vi "Dashboard Main.vi"() -> ()   [LabVIEW 2014]
uses:
  <vilib>/Rock Robotics/WPI/Dashboard/WPI_DashboardLogging Global.vi
  <vilib>/Utility/config.llb/NI_LVConfig.lvlib
  <vilib>/Utility/config.llb/Write Key (I32).vi
  Common Code/Utilities/PDP Data.ctl
  Common Code/commandCluster.ctl
  Common Code/AutonomousDBPacket.ctl
  Common Code/Roller Mode Enum.ctl
  Common Code/Auto Roller Commands.ctl
  Common Code/Roller Indicators.ctl
  Common Code/Elevator State.ctl
  Common Code/Elevator Status.ctl
  Common Code/Dashboard Display Data.ctl
  <vilib>/Utility/miscctls.llb/LVPointTypeDef.ctl
  Common Code/IMU Data.ctl
  Common Code/Inner Roller States.ctl
  Common Code/Elevator Mode.ctl
  Common Code/Encoder Values.ctl
  Common Code/Encoder Values SuperCluster.ctl
  Common Code/Utilities/PCM Data.ctl
  Common Code/Power and Diagnostic Data.ctl
  Common Code/Loop Timings.ctl
  Common Code/Ultrasonic Indicators.ctl
  Robot Code/Sensors/Pot Data.ctl
  Robot Code/Drivetrain Code/Drivetrain Mode.ctl
  Common Code/Drivetrain Status.ctl
  Robot Code/Rollers/ThinRollerIndicators.ctl
  Common Code/Auto Elevator Indicators.ctl
  Common Code/Dist Drive Status.ctl
  Common Code/Drivetrain Settings.ctl
  Common Code/Encoder Control.ctl
  Common Code/Elevator Presets.ctl
  Common Code/Elevator DB Control.ctl
  Common Code/Roller Control.ctl
  Common Code/Dashboard Control Data.ctl
  navX-MXP Library/COMMON/TypeDefs/Value TypeDefs/navX NAVX_OP_STATUS.ctl
  navX-MXP Library/navX-MXP IMU.lvlib
  navX-MXP Library/COMMON/TypeDefs/Value TypeDefs/navX NAVX_CAL_STATUS.ctl
  Robot Code/Rollers/Untip Can States.ctl
  Common Code/Yaw Rate Compensation Indicators.ctl
  Robot Code/Pike/Pike DB Controls.ctl
  Robot Code/Pike/Pike Mode.ctl
  Robot Code/Pike/Pike State.ctl
  Robot Code/Pike/Pike Indicators.ctl
  Common Code/Elevator Idle Mode.ctl
  Robot Code/Elevator/Elevator Command.ctl
  Robot Code/Elevator/Elevator Control Command.ctl
  <vilib>/Utility/inputDevices.llb/keyboardAcquire.vi
  <vilib>/Utility/config.llb/Write Key (String).vi
  <vilib>/Rock Robotics/WPI/Camera/WPI_CameraImageSize.ctl
  <vilib>/Rock Robotics/WPI/Camera/WPI_CameraSettings Read MJPG.ctl
  Vision/Particle Filter Settings.ctl
  <vilib>/vision/Image Controls.llb/IMAQ Image.ctl
  Vision/Vision Tote Data.ctl
panel:
  out "Axis Cam":T1
  out "DumbDash Message":string
  in  "Load":bool
  in  "Save":bool
  in  "stop":bool
  in  "TCP":refnum<k5>
  in  "Rec Mode":enum32{"Stop", "Record", "Playback"}(radio)
  out "Camera IP":string
  out "Image Message":string="Timeout in Camera Communications"
  in  "Dashboard Tab":T2(tab)
  out "2D Picture":picture
  in  "Useless Button":bool
  out "Elev Limit":bool
  out "Eject":bool
  out "Stabilizer":bool
  out "Finger":bool
  out "NAVX_CAL_STATUS":T3 items=["IMU_CAL_STATE_MASK"=3, "IMU_CAL_INPROGRESS"=0, "IMU_CAL_ACCUMULATE"=1, "IMU_CAL_COMPLETE"=2, "MAG_CAL_COMPLETE"=4, "BARO_CAL_COMPLETE"=8]
  out "Trashcan? 2":bool caption="Trashcan?"
  out "Robot Mode":T4(ring)=enum."Auto Disabled"
  out "Gyro":dbl(knob) scale=0.0..360.0 scale format="%#.7g"
  out "Elevator Mode":bool
  out "Roller Mode":bool
  out "Pressure":dbl format="%#.1f"
  out "Ultrasonic Data 2":T5
  out "Auton File":string
  out "Elevator Status Data 2":T6 {"Finger Raw" format="%#.3f"; "Finger Height" format="%#.3f"; "Motor Out" scale=-1.0..1.0}
  out "Robot IP":string
  out "Roller Indicators Thin":T10={"Rollers Closed?"=FALSE, "Roller Mode"=enum."Manual", "Left Out"=0.0, "Right Out"=0.0, "L Current"=1.0, "R Current"=1.0} {"Right Out" scale=-1.0..1.0; "Left Out" scale=-1.0..1.0}
  out "Elev Command":T12
  out "Idle Mode":T13
  out "Auton File Count":i32
  out "Directory":string
  out "Current File":string
  out "File Index":i32
  out "Current Auto Command Data":T14
  out "Drivetrain 4":T15 {"Translation X" scale=-1.0..1.0; "X (Steer)" scale=-1.0..1.0; "Y (Throttle)" scale=-1.0..1.0}
  in  "Mask View":bool
  in  "Camera Settings":T19={"Frame Rate"=30, "Compression"=30, "Size"=1} {"Frame Rate" scale=1.0..30.0; "Size" items=["640x480", "320x240", "160x120"]}
  in  "Camera FOV width":dbl
  in  "Cam Exposure":dbl
  out "Axis Display":T1(plugin-control)
  in  "Vision":u16(ring) items=["Camera Off", "USB Camera SW", "USB Camera HW", "IP Camera"]
  out "Mbps 2":bool
  out "Mbps":dbl format="%#.1g"
  out "fps":dbl format="%#.1g"
  in  "DB Camera Config":bool
  in  "File Path":path
  in  "Use File":bool
  in  "Min target size %":dbl format="%#_13g"
  in  "Camera Settings 2":T20={"fps"=30, "compression"=30, "Image Size"=enum."320x240"}
  out "USB Cam":T1(plugin-control)
  out "fps 2":dbl format="%#.1g"
  out "Mbps 2":dbl format="%#.1g"
  out "Total mbps":dbl
  in  "Filter Settings":T22
  in  "Ring Light Color":T23={"Hue"={101.37467765958063, 64.10933859299683}, "Sat"={88.03571428571429, 255.0}, "Val"={133.57142857142858, 255.0}} {"Hue" scale=0.0..255.0 scale format="%#_3g"}
  out "Detected totes":T24[](array[typedef])
  in  "Camera Mode":u16(ring) items=["Camera Off", "USB Camera SW", "USB Camera HW", "IP Camera"]
  in  "Rectangle":T25
  out "Power and Diagnostic Data":T26
  out "Status Info":T29
  out "Robot Metrics":T30
  out "DS TCP":T31
  out "Control Info":T32
  out "Loop Timings":T33
  out "IMU Gyro":dbl(knob) scale=0.0..360.0 scale format="%#.7g"
  out "Roll":dbl(knob) scale=-90.0..90.0
  out "Pitch":dbl(knob) scale=-90.0..90.0
  in  "Yaw PID Gains":T34={"proportional gain (Kc)"=0.0624, "integral time (Ti, min)"=0.0, "derivative time (Td, min)"=0.002}
  in  "Yaw PID Output Range":cluster{"output high":dbl, "output low":dbl}={"output high"=0.75, "output low"=-0.75}
  in  "Go to angle":dbl
  out "IMU Data":T35 {"NAVX_OP_STATUS" items=["INITIALIZING", "SELFTEST_IN_PROGRESS", "ERROR", "IMU_AUTOCAL_IN_PROGRESS", "NORMAL"]; "NAVX_CAL_STATUS" items=["IMU_CAL_STATE_MASK"=3, "IMU_CAL_INPROGRESS"=0, "IMU_CAL_ACCUMULATE"=1, "IMU_CAL_COMPLETE"=2, "MAG_CAL_COMPLETE"=4, "BARO_CAL_COMPLETE"=8]}
  in  "Drivetrain Settings":T37={"Gyro Tolerance"=0.0, "Strafe Correct max steer"=0.4, "Strafe Timer Wait"=250.0, "Throttle Ramp (ms)"=0.0, "Strafe Ramp (ms)"=0.0, "Angular rate compensation"=FALSE, "Throttle to Rate Scale"=0.0, "Rate compensation gain"=0.0, "Creep Steer"=0.0, "Creep Throttle"=0.0} {"Rate compensation gain" format="%#_6f"; "Throttle to Rate Scale" format="%#_6f"}
  out "Encoder Values":T38 {"Right Encoder"."Ticks" format="%#.6g"; "Center Encoder"."Ticks" format="%#.6g"; "Left Encoder"."Ticks" format="%#.6g"}
  in  "Encoder Control":T40={"Left Tick Constant"=1.0, "Right Tick Constant"=0.0, "Center Tick Constant"=0.0, "Reset?"=FALSE, "Y Dist"={"PID gains"={"proportional gain (Kc)"=1.0, "integral time (Ti, min)"=0.0, "derivative time (Td, min)"=0.0}}, "X Dist"={"PID gains"={"proportional gain (Kc)"=1.0, "integral time (Ti, min)"=0.0, "derivative time (Td, min)"=0.0}}, "Y Stop Thresh"=0.0, "Y Stop Speed"=0.0, "X Stop Thresh"=0.0, "X Stop Speed"=0.0} {"X Dist"."PID gains"."derivative time (Td, min)" format="%.6f"; "X Dist"."PID gains"."integral time (Ti, min)" format="%.6f"; "X Dist"."PID gains"."proportional gain (Kc)" format="%.6f"; "Y Dist"."PID gains"."derivative time (Td, min)" format="%.6f"; "Y Dist"."PID gains"."integral time (Ti, min)" format="%.6f"; "Y Dist"."PID gains"."proportional gain (Kc)" format="%.6f"}
  out "Drivetrain":T15 {"Translation X" scale=-1.0..1.0; "X (Steer)" scale=-1.0..1.0; "Y (Throttle)" scale=-1.0..1.0}
  out "Zeroing Rollers?":bool
  out "Roller State Indicators":T41={"Rollers Closed?"=FALSE, "Roller Mode"=enum."Manual", "Auto Roller State"=enum."Grab Tote", "Tote Inside?"=FALSE, "Intake State"=enum."Acquire Tote", "Left Ping Dist"=0.0, "Right Ping Dist"=0.0, "Potentiometer Cluster"={"Left Pot Zero"=0.0, "Right Pot Zero"=0.0, "Left Potentiometer"=0.0, "Right Potentiometer"=0.0, "Left Pot Non Zero"=0.0, "Right Pot Non Zero"=0.0}, "PING Decision"=enum."Acquire Tote", "Left Arm Closed?"=FALSE, "Portrait?"=FALSE, "Right Arm Closed?"=FALSE, "Left Out"=0.0, "Right Out"=0.0, "Left Current"=0.0, "Right Current"=0.0, "Tote Load Complete?"=FALSE, "Untip Complete?"=FALSE, "Untip State"=enum."Idle", "Roller Safety Open"=FALSE} {"Right Out" scale=-1.0..1.0; "Left Out" scale=-1.0..1.0}
  in  "Roller Settings":T46={"Intake Speed"=0.7, "Turn In Speed"=0.7, "Unload Speed"=-0.7, "Turn Out Speed"=-0.7, "Ping Align Tolerance"=1000.0, "Tote Range Threshold"=0.0, "Right Pot 0"=0.0, "Pot Threshold"=0.0, "Left Pot 0"=0.0, "Right Pot Scale"=0.0, "Left Pot Scale"=0.0, "Min Elevator Height"=0.0, "Eject Time"=0.0, "Eject US Threshold"=0.0, "Anti-Twitch Time"=0, "Ping Caring Threshold"=0.0, "Pot Diff Threshold"=0.0, "Pinch Sustain"=0, "Absorb Give Up Threshold"=0.0, "Untip In Threshold"=0.0, "Untip Grab Range"=0.0, "Ultrasonic Hold Time"=0, "Landscape Absorb Time"=0, "Pot Use Wait Time"=0, "Can Turn Stop Range"=0.0, "HP Load Speed"=0.0, "Stick Multiplier"=0.0, "Coop Eject Speed"=0.0}
  out "Ultrasonic Data":T5
  in  "Pressure m Value":dbl=34.774
  in  "Pressure b Value":dbl=-58.564
  out "Transducer Voltage":dbl
  out "Pressure 2":dbl
  out "Trashcan?":bool
  in  "Elevator":T47={"PID Output Range"={"output high"=1.0, "output low"=-1.0}, "PID gains"={"proportional gain (Kc)"=1.0, "integral time (Ti, min)"=0.0, "derivative time (Td, min)"=0.0}, "Height Tolerance"=0.5, " Encoder Constant"=0.0027952480782669, "Eject Time"=0.0, "Zeroing Speed"=1.0, "Presets"={"Pickup 2 w/ Tote"=27.0, "Pickup 2 w/ Trashcan"=25.0, "Pickup 3 w/ Tote"=40.0, "Pickup 3 w/ Trashcan"=25.0, "Bottom"=0.0, "Pickup 1 w/ Tote"=17.0, "Pickup Trashcan"=0.0, "Pickup 1 w/ Trashcan"=25.0, "Eject"=0.0, "Hold Low"=0.0, "Step add height"=0.0, "Untip Lift"=0.0, "Drop Stack"=0.0, "HP Load Hold"=0.0, "HP Load Drop"=0.0, "HP Load Hold Can"=0.0, "Store can max"=0.0, "HP Drag Score"=0.0, "HP Drag Finish"=0.0, "Finger trashcan avoid"=0.0, "Full"=0.0}, "Ping Detect Threshold"=0.0, "Trashcan Detect Threshold"=0.0, "Zero Filter Time"=0.0, "Stabilizer Open Time"=0.0, "Zero Creep Speed"=0.0, "Max Current"=0.0, "Current Trip Time"=0.0, "Abort Pitch"=0.0, "Finger m"=0.0, "Finger b"=0.0, "Finger max "=0.0, "Finger Stabilizer"=0.0, "Finger Store"=0.0, "Finger Stop Store"=0.0, "Stabilizer Close Time"=0.0, "Finger min"=0.0, "Unstick gain"=0.0, "Full Detect Max"=0.0} {"Encoder Constant" format="%.6f"}
  out "Ultrasonic Data 3":T5
  out "Elevator Status Data 3":T6 {"Motor Out" scale=-1.0..1.0}
  out "Elevator Command":T49={"Command"=enum."Idle", "Manual Motor Out"=0.0, "Manual Eject Piston"=FALSE, "Mode"=enum."Manual", "Override Limits"=FALSE, "Manual Stabilizer"=FALSE, "Manual Finger"=FALSE, "Store Trashcan?"=FALSE, "Hold Low?"=FALSE, "Idle Mode"=enum."Load Can", "HP Load"=FALSE, "Unstick"=FALSE, "Raw Height Set"=0.0, "Force Store"=FALSE}
  in  "OH BABY A TRIPLE":bool
  out "2D Picture 2":picture
  # "Steering PID"
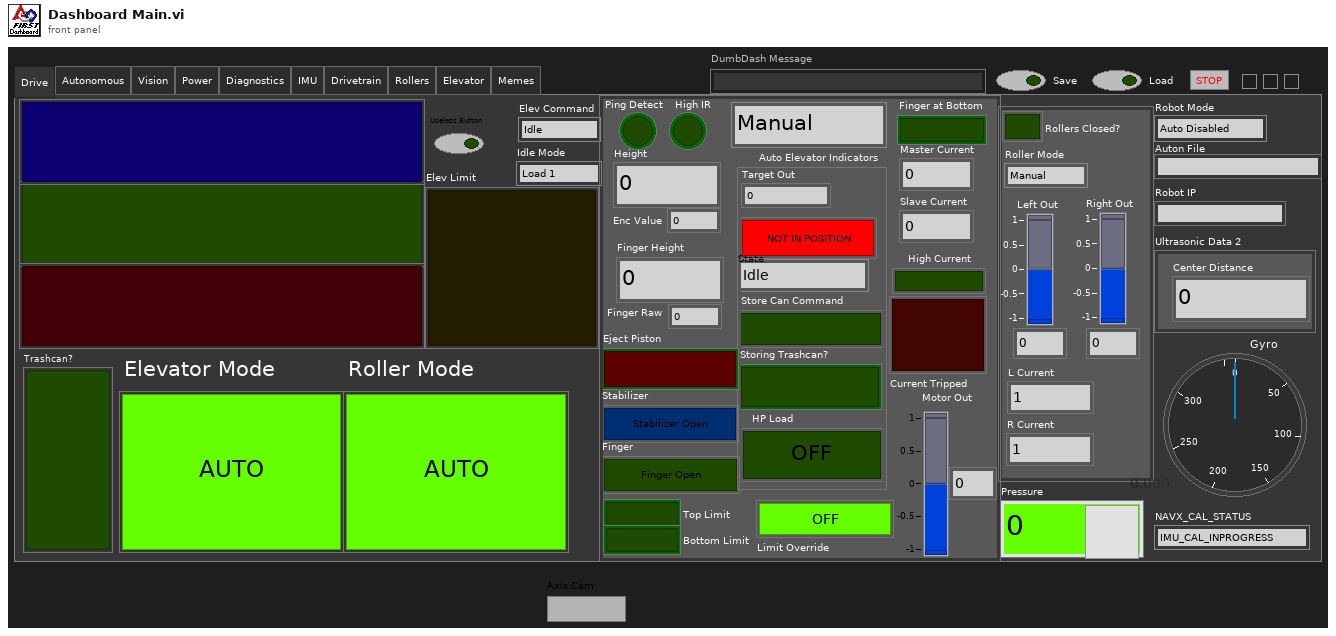
[diagram p1: front panel]
types:
  T1 = typedef "IMAQ Image.ctl" = refnum<image>
  T2 = enum32{"Drive", "Autonomous", "Vision", "Power", "Diagnostics", "IMU", "Drivetrain", "Rollers", "Elevator", "Memes"}
  T3 = typedef "navX-MXP IMU.lvlib/navX NAVX_CAL_STATUS.ctl" = u8
  T4 = enum8{"Tele-Op Disabled", "Tele-Op Enabled", "Auto Disabled", "Auto Enabled", "Test Disabled", "Test Enabled", "Disconnected", "No Code", "E-Stop"}
  T5 = typedef "Ultrasonic Indicators.ctl" = cluster{"Left Distance":dbl, "Right Distance":dbl, "Center Distance":dbl, "Left Distance Unfilter":dbl, "Right Distance Unfilter":dbl, "Center Distance Unfilter":dbl}
  T6 = typedef "Elevator Status.ctl" = cluster{"Height":dbl, "Enc Value":dbl, "Limit Override":bool, "Mode":T7, "High IR":bool, "Motor Out":dbl, "Ping Detect":bool, "Auto Elevator Indicators":T8, "Master Current":dbl, "Slave Current":dbl, "High Current":bool, "Current Tripped":bool, "Top Limit":bool, "Bottom Limit":bool, "Eject Piston":bool, "Stabilizer":bool, "Finger":bool, "Finger Height":dbl, "Finger Raw":dbl, "Finger at Bottom":bool}
  T7 = typedef "Elevator Mode.ctl" = enum16{"Manual", "Safe", "Auto"}
  T8 = typedef "Auto Elevator Indicators.ctl" = cluster{"Target Out":dbl, "Storing Trashcan?":bool, "State":T9, "In Range":bool, "Store Can Command":bool, "HP Load":bool}
  T9 = typedef "Elevator State.ctl" = enum16{"Idle", "Goto Load Position", "Wait for Load", "Load Drop", "Load Lift", "Drop Stack", "Goto Eject Position", "Eject ", "Raise Trashcan", "Open Stabilizer", "Untip Drop", "Untip Wait", "Untip Lift", "Abort Load", "HP Load Wait", "HP Load Drop", "HP Load Lift", "HP Load Abort", "Close Stabilizer", "HP Load Unfinish", "HP Load Score", "HP Load Finish", "HP Goto Finish Down", "HP Goto Finish Up", "Full"}
  T10 = typedef "ThinRollerIndicators.ctl" = cluster{"Rollers Closed?":bool, "Roller Mode":T11, "Left Out":dbl, "Right Out":dbl, "L Current":dbl, "R Current":dbl}
  T11 = typedef "Roller Mode Enum.ctl" = enum16{"Manual", "Safe", "Auto"}
  T12 = typedef "Elevator Command.ctl" = enum16{"Idle", "Load 1", "Load 2", "Load 3", "Drop Stack", "Eject Stack", "Untip Trashcan", "Load Trashcan", "HP Load", "HP Score"}
  T13 = typedef "Elevator Idle Mode.ctl" = enum16{"Load 1", "Load 2", "Load 3", "Load Can", "Untip Can", "Step Load", "Drop Stack", "Raw Height"}
  T14 = typedef "commandCluster.ctl" = cluster{"Step ID":i16, "Command Type":i16, "Drive X":sgl, "Drive Y":sgl, "Heading":sgl, "Max Exec. Time":i16, "Jump Type":i32, "Jump To":i16, "Jump Condition":i16, "Async Drive?":i16, "Roller Mode":i16, "Roller Align":i16, "Roller Closed?":i16, "Wait Condition":i16, "Elevator Mode":i16, "Elevator Command":i16, "Roller State":i16, "Hold Low?":i16, "Num Totes":i16, "Num Cans":dbl, "Past Distance":dbl, "Store Can?":dbl, "X Speed":dbl, "Y Speed":dbl, "Yaw Angle Set":dbl, "Grab Can":dbl, "Roller Overide Speed":dbl, "Force Load?":sgl, "Set Idle":sgl, "Eject":sgl, "Pike Action":sgl, "Pivot Speed":dbl, "Height":dbl}
  T15 = typedef "Drivetrain Status.ctl" = cluster{"Y (Throttle)":sgl, "X (Steer)":sgl, "Translation X":sgl, "Center Wheel Down":bool, "Mode":T16, "Distance Drive finished?":bool, "Y Target":sgl, "X Target":sgl, "Heading Target":sgl, "Dist Drive Status":T17, "Step Eject Lockout":bool, "Gyro In Range?":bool, "Yaw Comp Indicators":T18}
  T16 = typedef "Drivetrain Mode.ctl" = enum16{"Manual", "Gyro Steer", "Vision Steer", "Drive Distance", "Yaw Rate Compensate"}
  T17 = typedef "Dist Drive Status.ctl" = cluster{"Y In Range":bool, "X In Range":bool, "Gyro In Range":bool, "Y Dist":dbl, "X Dist":dbl, "Gyro":dbl}
  T18 = typedef "Yaw Rate Compensation Indicators.ctl" = cluster{"Rate Command":sgl, "Rate Actual":sgl, "Steer adjustment":sgl}
  T19 = cluster{"Frame Rate":i32, "Compression":i32, "Size":u16}
  T20 = typedef "WPI_CameraSettings Read MJPG.ctl" = cluster{"fps":i32, "compression":i32, "Image Size":T21}
  T21 = typedef "WPI_CameraImageSize.ctl" = enum16{"640x480", "320x240", "160x120", "Custom"}
  T22 = typedef "Particle Filter Settings.ctl" = cluster{"Min Aspect Score":dbl, "Min Area Score":dbl, "Min X Score":dbl, "Min Y Score":dbl}
  T23 = cluster{"Hue":cluster{dbl, dbl}, "Sat":cluster{dbl, dbl}, "Val":cluster{dbl, dbl}}
  T24 = typedef "Vision Tote Data.ctl" = cluster{"Left _|":cluster{"Bounding box":cluster{"left":dbl, "top":dbl, "right":dbl, "bottom":dbl}, "Aspect Ratio":dbl, "Area Score":dbl, "X Mask":dbl, "Y Mask":dbl, "Ell":bool}, "Right |_":cluster{"Bounding box":cluster{"left":dbl, "top":dbl, "right":dbl, "bottom":dbl}, "Aspect Ratio":dbl, "Area Score":dbl, "X Mask":dbl, "Y Mask":dbl, "Ell":bool}, "Center X":dbl, "Center Y":dbl, "Angle Offset":dbl}
  T25 = cluster{"Left":i32, "Top":i32, "Right":i32, "Bottom":i32}
  T26 = typedef "Power and Diagnostic Data.ctl" = cluster{"PDP Data":T27, "PCM Data":T28, "roboRIO input voltage (V)":dbl, "roboRIO input current (A)":dbl, "3.3V Rail Short":bool, "5 V Rail Short":bool, "6 V Rail Short":bool, "roboRIO Brownout":bool, "Outputs Enabled?":bool}
  T27 = typedef "PDP Data.ctl" = cluster{"Battery Voltage":sgl, "Temperature (degrees C)":sgl, "Internal Battery R (Ohms)":sgl, "Energy (J)":sgl, "Power (W)":sgl, "Total Current (A)":sgl, "Battery Voltage Fault":bool, "Temperature Fault":bool, "Hardware Fault":bool, "Currents":cluster{"[0]":sgl, "[1]":sgl, "[2]":sgl, "[3]":sgl, "[4]":sgl, "[5]":sgl, "[6]":sgl, "[7]":sgl, "[8]":sgl, "[9]":sgl, "[10]":sgl, "[11]":sgl, "[12]":sgl, "[13]":sgl, "[14]":sgl, "[15]":sgl}, "Current Faults":cluster{"[0]":bool, "[1]":bool, "[2]":bool, "[3]":bool, "[4]":bool, "[5]":bool, "[6]":bool, "[7]":bool, "[8]":bool, "[9]":bool, "[10]":bool, "[11]":bool, "[12]":bool, "[13]":bool, "[14]":bool, "[15]":bool}}
  T28 = typedef "PCM Data.ctl" = cluster{"Compressor Fault":bool, "Solenoid Fault":bool, "Compressor Enabled":bool, "Hardware Fault":bool, "Compressor Current":dbl}
  T29 = cluster{"Status bits":cluster{"Test Mode":bool, "Autonomous":bool, "Enabled":bool, "Code Start":bool, "Brownout":bool, "Reserved 2":bool, "Reserved 3":bool, "E-Stop":bool}, "Code Trace":cluster{"Disabled":bool, "TeleOp":bool, "Auto":bool, "Test":bool}, "Controller Type":enum16{"unknown", "cRIO", "roboRio"}, "Code?":enum16{"unknown", "noCode", "code"}, "Battery V":dbl}
  T30 = cluster{"Storage":cluster{"Disk Free":u64, "RAM Block":u32, "RAM free":u32}, "CPU Utilization":cluster{"CPU % ISR":sgl, "CPU % Time Crit":sgl, "CPU % Timed Str":sgl, "CPU % High":sgl, "CPU % Above":sgl, "CPU % Normal":sgl, "CPU % Low":sgl}, "CAN":cluster{"% Bus Utilization":sgl, "Bus Off Cnt":u32, "TX_FIFO Full Cnt":u32, "Receive Error Cnt":u8, "Transmit Error Cnt":u8}, "HID":cluster{"HID Outputs":u32, "Rumble Low":u16, "Rumble High":u16}[]}
  T31 = cluster{"Error Strings":string, "Disable Counts":cluster{u16, u16}, "Rail Faults":cluster{u16, u16, u16}, "Robot IP":string, "DB Mode":u8, "Event Info":cluster{"Name":string, "Type":u8, "Number":u16, "Replay":u8}, "Camera Addr":string}
  T32 = cluster{"Control Bits":cluster{"TestMode":bool, "Autonomous":bool, "Enabled":bool, "FMS Present":bool, bool, bool, bool, "E-Stop":bool}, "Team Station ":u8, "Countdown":sgl, "Joystick Values":cluster{"Axes":dbl[], "Buttons":bool[], "POVs":i16[]}[]}
  T33 = typedef "Loop Timings.ctl" = cluster{"Roller Loop":i32, "Elevator Loop":i32, "US Loop":i32, "100ms Loop":i32, "Drivetrain Loop":i32}
  T34 = cluster{"proportional gain (Kc)":dbl, "integral time (Ti, min)":dbl, "derivative time (Td, min)":dbl}
  T35 = typedef "IMU Data.ctl" = cluster{"Pitch":sgl, "Roll":sgl, "Yaw":sgl, "Data Valid?":bool, "Temp":sgl, "MOVING":bool, "NAVX_CAL_STATUS":T3, "NAVX_OP_STATUS":T36, "YAW_STABLE":bool, "Accel X":sgl, "Accel Y":sgl, "Accel Z":sgl, "Accel Magnitude":sgl, "Pitch Rate":sgl, "Roll Rate":sgl, "Yaw Rate":sgl, "NavX Opened?":bool}
  T36 = typedef "navX-MXP IMU.lvlib/navX NAVX_OP_STATUS.ctl" = u8
  T37 = typedef "Drivetrain Settings.ctl" = cluster{"Gyro Tolerance":sgl, "Strafe Correct max steer":sgl, "Strafe Timer Wait":sgl, "Throttle Ramp (ms)":sgl, "Strafe Ramp (ms)":sgl, "Angular rate compensation":bool, "Throttle to Rate Scale":sgl, "Rate compensation gain":sgl, "Creep Steer":sgl, "Creep Throttle":sgl}
  T38 = typedef "Encoder Values SuperCluster.ctl" = cluster{"Left Encoder":T39, "Center Encoder":T39, "Right Encoder":T39}
  T39 = typedef "Encoder Values.ctl" = cluster{"Distance":dbl, "Speed":dbl, "Ticks":dbl}
  T40 = typedef "Encoder Control.ctl" = cluster{"Left Tick Constant":dbl, "Right Tick Constant":dbl, "Center Tick Constant":dbl, "Reset?":bool, "Y Dist":cluster{"PID gains":cluster{"proportional gain (Kc)":dbl, "integral time (Ti, min)":dbl, "derivative time (Td, min)":dbl}}, "X Dist":cluster{"PID gains":cluster{"proportional gain (Kc)":dbl, "integral time (Ti, min)":dbl, "derivative time (Td, min)":dbl}}, "Y Stop Thresh":dbl, "Y Stop Speed":dbl, "X Stop Thresh":dbl, "X Stop Speed":dbl}
  T41 = typedef "Roller Indicators.ctl" = cluster{"Rollers Closed?":bool, "Roller Mode":T11, "Auto Roller State":T42, "Tote Inside?":bool, "Intake State":T43, "Left Ping Dist":sgl, "Right Ping Dist":sgl, "Potentiometer Cluster":T44, "PING Decision":T43, "Left Arm Closed?":bool, "Portrait?":bool, "Right Arm Closed?":bool, "Left Out":sgl, "Right Out":sgl, "Left Current":sgl, "Right Current":sgl, "Tote Load Complete?":bool, "Untip Complete?":bool, "Untip State":T45, "Roller Safety Open":bool}
  T42 = typedef "Auto Roller Commands.ctl" = enum16{"Drag Tote", "Grab Tote", "Idle", "Eject Tote", "Untip Can", "Grab Can"}
  T43 = typedef "Inner Roller States.ctl" = enum16{"Turn Tote Portrait", "Acquire Tote", "Absorb Tote", "Turn Tote Right", "Turn Tote Left", "Acquire Can", "Absorb Can", "Turn Can", "Hold Tote"}
  T44 = typedef "Pot Data.ctl" = cluster{"Left Pot Zero":sgl, "Right Pot Zero":sgl, "Left Potentiometer":sgl, "Right Potentiometer":sgl, "Left Pot Non Zero":sgl, "Right Pot Non Zero":sgl}
  T45 = typedef "Untip Can States.ctl" = enum16{"Release Can", "Catch Can", "Idle"}
  T46 = typedef "Roller Control.ctl" = cluster{"Intake Speed":dbl, "Turn In Speed":dbl, "Unload Speed":dbl, "Turn Out Speed":dbl, "Ping Align Tolerance":dbl, "Tote Range Threshold":dbl, "Right Pot 0":dbl, "Pot Threshold":dbl, "Left Pot 0":dbl, "Right Pot Scale":dbl, "Left Pot Scale":dbl, "Min Elevator Height":dbl, "Eject Time":dbl, "Eject US Threshold":dbl, "Anti-Twitch Time":u32, "Ping Caring Threshold":dbl, "Pot Diff Threshold":dbl, "Pinch Sustain":u32, "Absorb Give Up Threshold":dbl, "Untip In Threshold":dbl, "Untip Grab Range":dbl, "Ultrasonic Hold Time":u32, "Landscape Absorb Time":u32, "Pot Use Wait Time":u32, "Can Turn Stop Range":dbl, "HP Load Speed":dbl, "Stick Multiplier":dbl, "Coop Eject Speed":dbl}
  T47 = typedef "Elevator DB Control.ctl" = cluster{"PID Output Range":cluster{"output high":dbl, "output low":dbl}, "PID gains":cluster{"proportional gain (Kc)":dbl, "integral time (Ti, min)":dbl, "derivative time (Td, min)":dbl}, "Height Tolerance":sgl, " Encoder Constant":dbl, "Eject Time":sgl, "Zeroing Speed":sgl, "Presets":T48, "Ping Detect Threshold":sgl, "Trashcan Detect Threshold":sgl, "Zero Filter Time":dbl, "Stabilizer Open Time":dbl, "Zero Creep Speed":dbl, "Max Current":dbl, "Current Trip Time":dbl, "Abort Pitch":dbl, "Finger m":dbl, "Finger b":dbl, "Finger max ":dbl, "Finger Stabilizer":dbl, "Finger Store":dbl, "Finger Stop Store":dbl, "Stabilizer Close Time":dbl, "Finger min":dbl, "Unstick gain":dbl, "Full Detect Max":dbl}
  T48 = typedef "Elevator Presets.ctl" = cluster{"Pickup 2 w/ Tote":sgl, "Pickup 2 w/ Trashcan":sgl, "Pickup 3 w/ Tote":sgl, "Pickup 3 w/ Trashcan":sgl, "Bottom":sgl, "Pickup 1 w/ Tote":sgl, "Pickup Trashcan":sgl, "Pickup 1 w/ Trashcan":sgl, "Eject":sgl, "Hold Low":sgl, "Step add height":sgl, "Untip Lift":dbl, "Drop Stack":dbl, "HP Load Hold":dbl, "HP Load Drop":dbl, "HP Load Hold Can":dbl, "Store can max":dbl, "HP Drag Score":dbl, "HP Drag Finish":dbl, "Finger trashcan avoid":dbl, "Full":dbl}
  T49 = typedef "Elevator Control Command.ctl" = cluster{"Command":T12, "Manual Motor Out":dbl, "Manual Eject Piston":bool, "Mode":T7, "Override Limits":bool, "Manual Stabilizer":bool, "Manual Finger":bool, "Store Trashcan?":bool, "Hold Low?":bool, "Idle Mode":T13, "HP Load":bool, "Unstick":bool, "Raw Height Set":dbl, "Force Store":bool}
  T50 = typedef "Image Type" = u32
  T51 = enum32{"Invalid", "Standard", "Closed", "Hidden", "Minimized", "Maximized"}
  T52 = typedef "LVPointTypeDef.ctl" = cluster{"Horizontal":i16, "Vertical":i16}
  T53 = typedef "Dashboard Display Data.ctl" = cluster{"Gyro Angle":dbl, "Autonomous":T54, "Pressure Transducer V":dbl, "Pressure":dbl, "Roller State Indicators":T41, "Elevator Status Data":T6, "IMU Data":T35, "Tote Count":i8, "Have Trashcan":bool, "Encoder Values":T38, "Power and Diagnostic Data":T26, "Loop Timings":T33, "Ultrasonic Data":T5, "Zeroing Rollers?":bool, "Drivetrain":T15, "Current Auto Command Data":T14, "Can Grabber":bool, "Pike":T55, "Elevator Command":T49}
  T54 = typedef "AutonomousDBPacket.ctl" = cluster{"Selected File":string, "Directory":string, "Auton File Index":i32, "Auton File Count":i32, "Auton Command Array":T14[]}
  T55 = typedef "Pike Indicators.ctl" = cluster{"Motor Out":dbl, "Current":dbl, "Limit Switch":bool, "Current Limit":bool, "State":T56, "Command":T57}
  T56 = typedef "Pike State.ctl" = enum16{"Up", "Down", "Going Up", "Going Down"}
  T57 = typedef "Pike Mode.ctl" = enum16{"Idle", "Auto Down", "Auto Up", "Manual Down", "Manual Up"}
  T58 = typedef "NI_LVConfig.lvlib/Config Data RefNum.ctl" = refnum<k1>
  T59 = typedef "Dashboard Control Data.ctl" = cluster{"Cam Exposure":dbl, "Go to angle":dbl, "Steer PID Gains":cluster{"proportional gain (Kc)":dbl, "integral time (Ti, min)":dbl, "derivative time (Td, min)":dbl}, "Steer PID output Range":cluster{"output high":dbl, "output low":dbl}, "Pressure m \nValue":dbl, "Pressure b \nValue":dbl, "Roller Command Cluster ":T46, "Elevator":T47, "Encoder Control":T40, "Auton Settings":cluster{"Drive Dist Window Size":dbl}, "Drivetrain Settings":T37, "Lance":T60}
  T60 = typedef "Pike DB Controls.ctl" = cluster{"Down Speed":dbl, "Up Speed":dbl, "Max Down Time":dbl, "Max Up Time":dbl, "Current Limit":dbl}
  T61 = cluster{"Image Size":bool, "Image Type":bool, "Pixel Value":bool, "ROI Information":bool, "Zoom Factor":bool}
  T62 = enum8{"Enabled", "Disabled", "Disabled and Grayed Out"}
  T63 = enum16{"0", "1", "2", "3", "4", "5", "6", "7", "8", "9", "A", "B", "C", "D", "E", "F", "G", "H", "I", "J", "K", "L", "M", "N", "O", "P", "Q", "R", "S", "T", "U", "V", "W", "X", "Y", "Z", "F1", "F2", "F3", "F4", "F5", "F6", "F7", "F8", "F9", "F10", "F11", "F12", "F13", "F14", "F15", "ADD", "BACK", "BACKSLASH", "CAPITAL", "COMMA", "DECIMAL", "DELETE", "DIVIDE", "DOWN", "END", "EQUALS", "ESCAPE", "GRAVE (`)", "HOME", "INSERT", "LBRACKET", "LCONTROL", "LEFT", "L ALT", "LSHIFT", "LWIN", "MINUS", "MULTIPLY", "NEXT", "NUMLOCK", "NUMPAD_0", "NUMPAD_1", "NUMPAD_2", "NUMPAD_3", "NUMPAD_4", "NUMPAD_5", "NUMPAD_6", "NUMPAD_7", "NUMPAD_8", "NUMPAD_9", "PAUSE", "PERIOD", "PRIOR (PG UP)", "RBRACKET", "RCONTROL", "RETURN", "RIGHT", "R ALT", "RSHIFT", "RWIN", "SCROLL", "SEMICOLON", "SLASH", "SPACE", "SUBTRACT", "TAB", "UP", "ENTER (num pad)", "' (quote)"}[]
  T64 = typedef "DumbDash Control.ctl" = cluster{"Name":string, "Ref":refnum<vi>, "Type":T65}
  T65 = typedef "DumbDash Control Type.ctl" = enum16{"Invalid", "Number", "Boolean", "String"}
  T66 = typedef "imagedata.ctl" = cluster{"image type":i32, "image depth":i32, "image":u8[], "mask":u8[], "colors":u32[], "Rectangle":cluster{"left":i16, "top":i16, "right":i16, "bottom":i16}}
  T67 = typedef "LVBoundsTypeDef.ctl" = cluster{"Width":u32, "Height":u32}
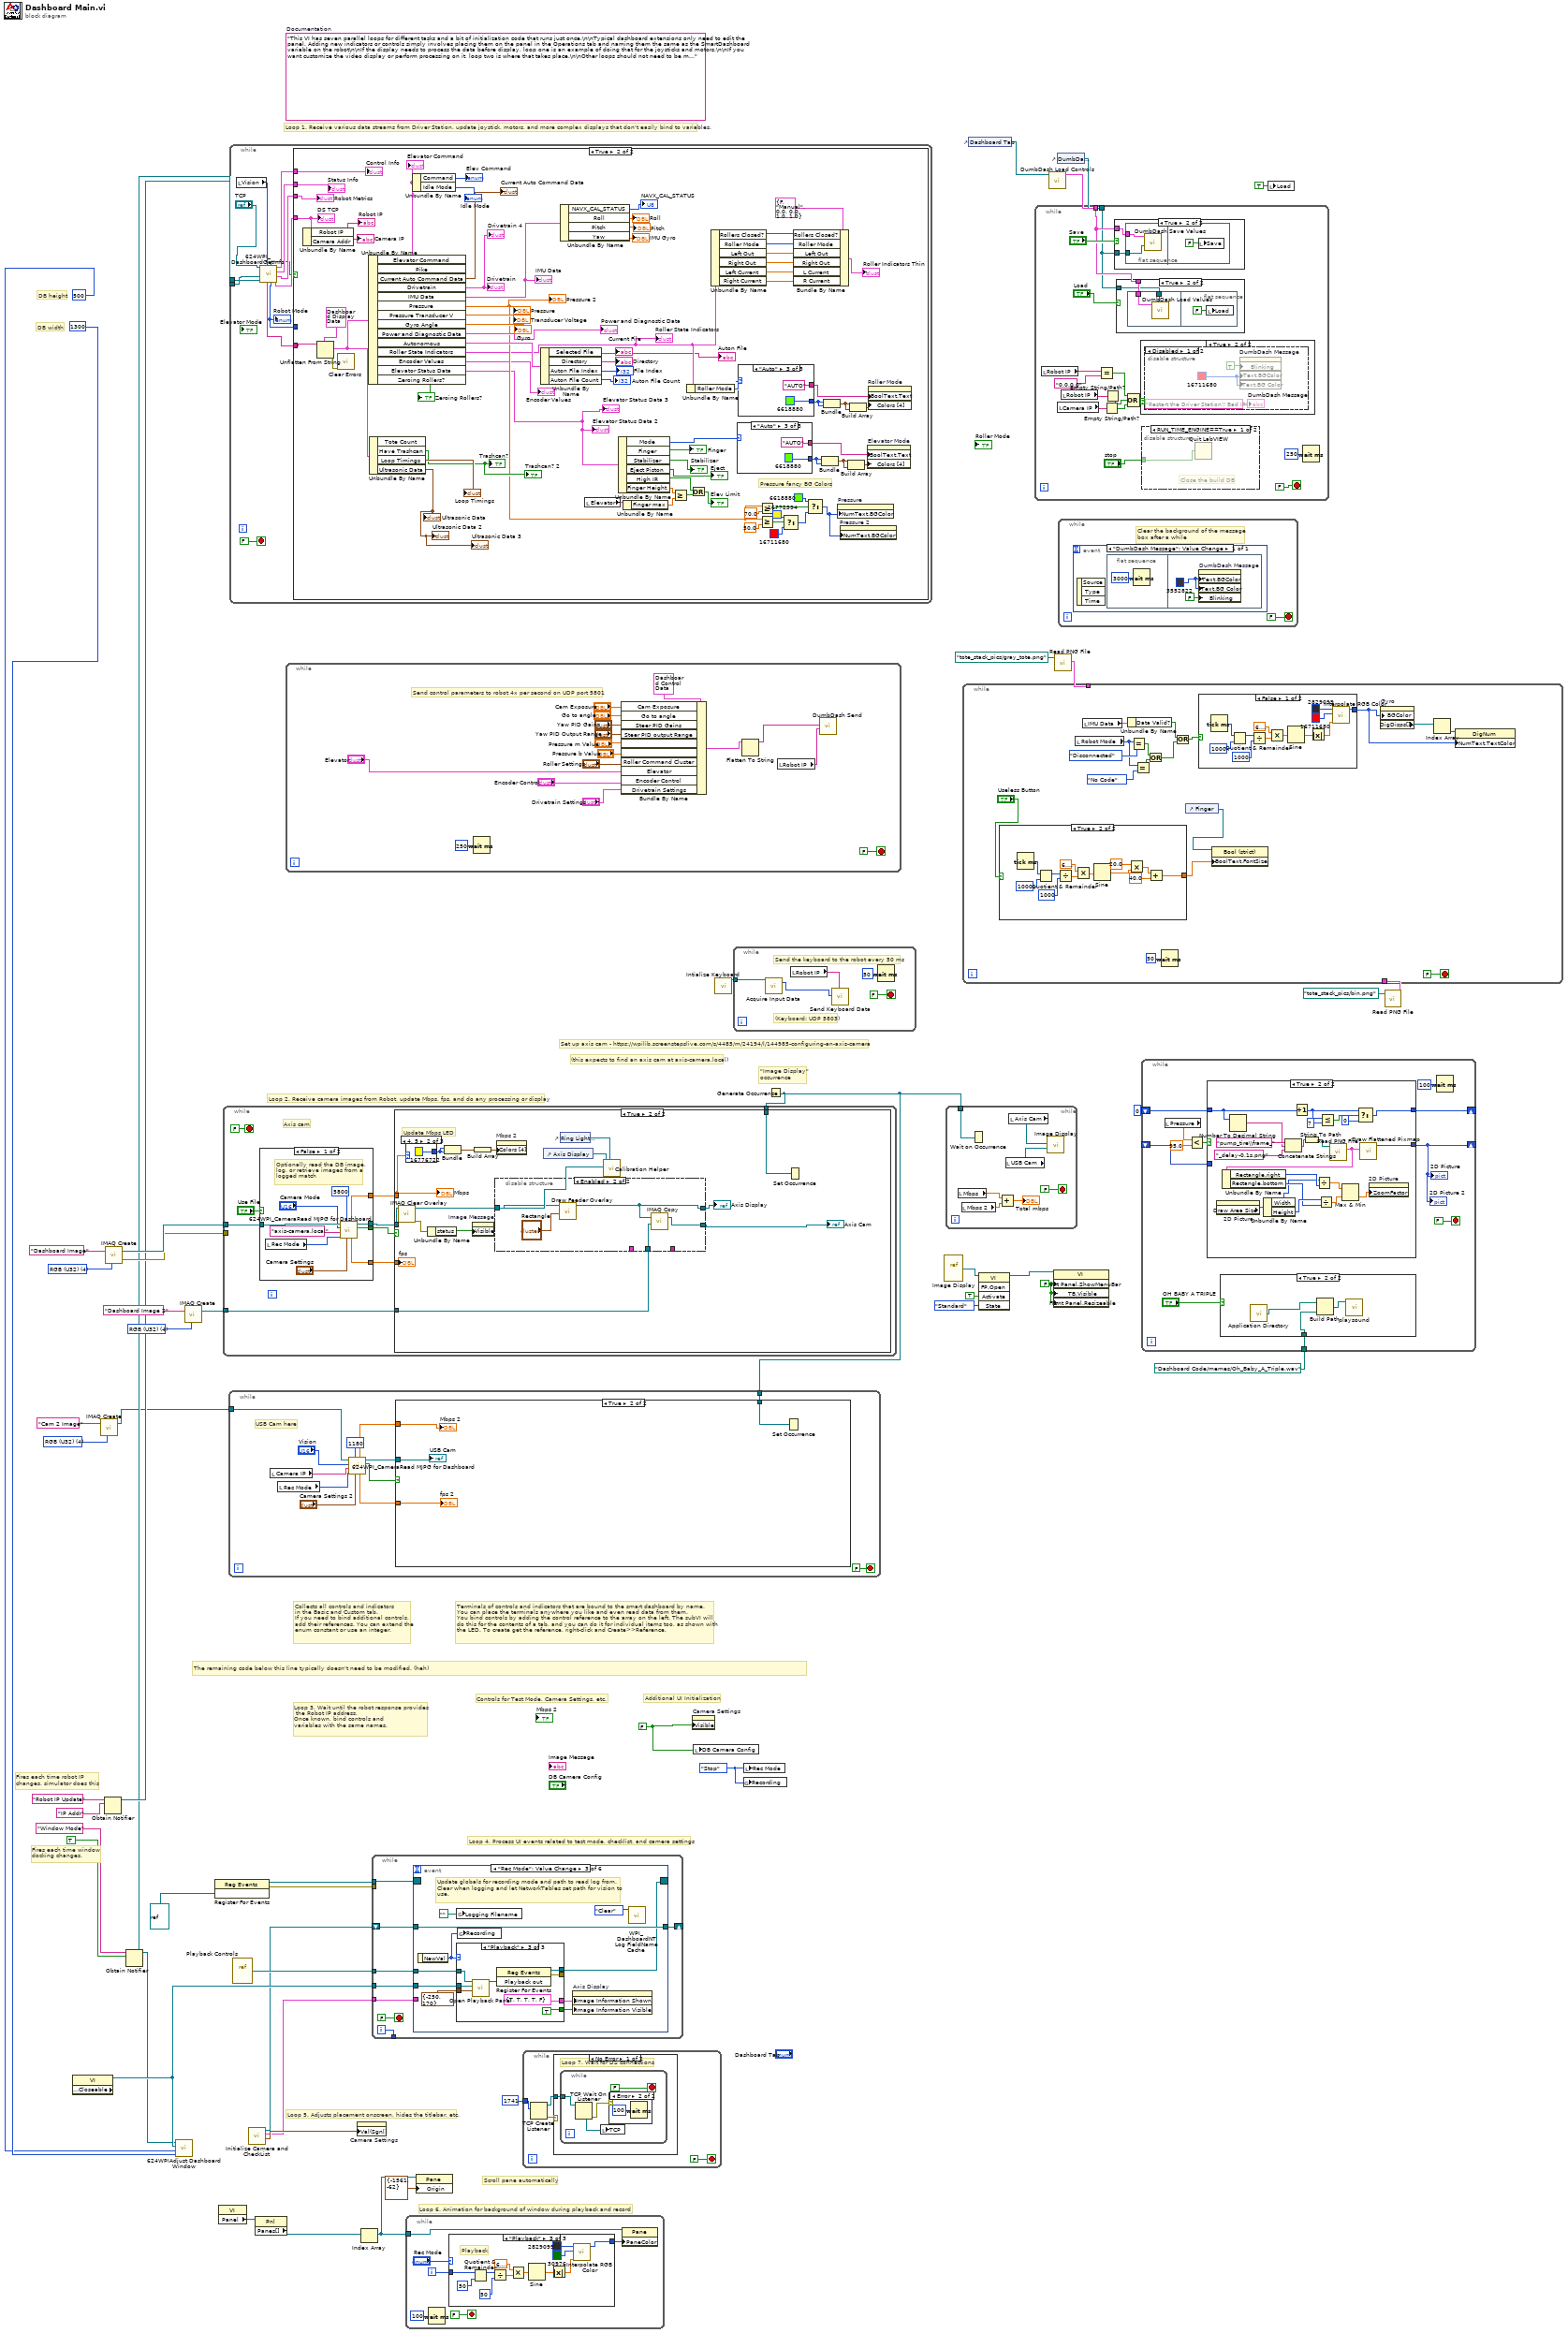
[diagram p0: block diagram]
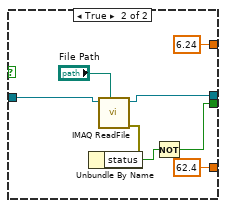
[diagram p2: hidden frame]
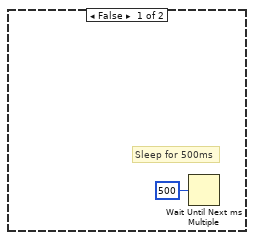
[diagram p3: hidden frame]
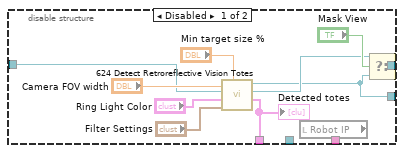
[diagram p4: hidden frame]
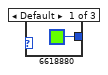
[diagram p5: hidden frame]
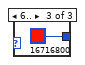
[diagram p6: hidden frame]
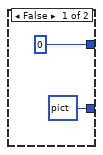
[diagram p8: hidden frame]
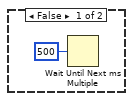
[diagram p11: hidden frame]
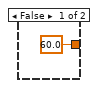
[diagram p12: hidden frame]
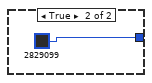
[diagram p13: hidden frame]
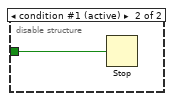
[diagram p14: hidden frame]
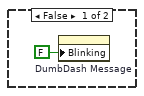
[diagram p15: hidden frame]
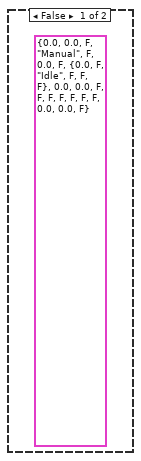
[diagram p19: hidden frame]
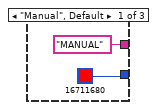
[diagram p20: hidden frame]
diagram:
  w5 = T50 4 items=["Grayscale (U8)", "Grayscale (I16)", "Grayscale (SGL)", "Complex (CSG)", "RGB (U32)", "HSL (U32)", "RGB (U64)"] ("Image Type")
  w8 = FALSE ("Front Panel Window:Show Menu Bar")
  w18 = T50 4 items=["Grayscale (U8)", "Grayscale (I16)", "Grayscale (SGL)", "Complex (CSG)", "RGB (U32)", "HSL (U32)", "RGB (U64)"] ("Image Type")
  w36 = enum32{"Stop", "Record", "Playback"}."Stop" ("Rec Mode")
  w34 = FALSE ("Visible")
  (unwired) "This VI has seven parallel loops for different tasks and a bit of initialization code that runs just once.\n\nTypical dashboard extensions only need to edit the panel. Adding new indicators or controls simply involves placing them on the panel in the Operations tab and naming them the same as the SmartDashboard variable on the robot\n\nIf the display needs to process the data before display, loop one is an example of doing that for the joysticks and motors.\n\nIf you want customize the video display or perform processing on it, loop two is where that takes place.\n\nOther loops should not need to be modified. They are pretty standard, and document the task they perform."  # Documentation
  w50 = T50 4 items=["Grayscale (U8)", "Grayscale (I16)", "Grayscale (SGL)", "Complex (CSG)", "RGB (U32)", "HSL (U32)", "RGB (U64)"] ("Image Type")
  # "\"Image Display\"\noccurrence"
  # "Loop 2. Receive camera images from Robot, update Mbps, fps, and do any processing or display"
  # "(this expects to find an axis cam at axis-camera.local)"
  # "Set up axis cam - https://wpilib.screenstepslive.com/s/4485/m/24194/l/144985-configuring-an-axis-camera"
  # "Scroll pane automatically"
  # "DB height"
  # "DB width"
  # "Controls for Test Mode, Camera Settings, etc."
  # "Additional UI Initialization"
  # "Loop 6. Animation for background of window during playback and record"
  # "Fires each time robot IP\nchanges, simulator does this"
  # "Fires each time window\ndocking changes."
  # "Collects all controls and indicators\nin the Basic and Custom tab.\nIf you need to bind additional controls,\nadd their references. You can extend the\nenum constant or use an integer."
  # "The remaining code below this line typically doesn't need to be modified. (heh)"
  # "Loop 4. Process UI events related to test mode, checklist, and camera settings"
  # "Terminals of controls and indicators that are bound to the smart dashboard by name.\nYou can place the terminals anywhere you like and even read data from them.\nYou bind controls by adding the control reference to the array on the left. The subVI will\ndo this for the contents of a tab, and you can do it for individual items too, as shown with\nthe LED. To create get the reference, right-click and Create>>Reference."
  # "Loop 3. Wait until the robot response provides\n the Robot IP address.\nOnce known, bind controls and\nvariables with the same names."
  # "Loop 5. Adjusts placement onscreen, hides the titlebar, etc."
  # "Loop 1. Receive various data streams from Driver Station, update joystick, motors, and more complex displays that don't easily bind to variables."
  n1 = property class="VI" props=["Front Panel.Closeable"]() -> (reference out=w35:refnum<vi>)  [unwired: 2 in, 2 out]
  n2 = call "IMAQ Create"("Image Name"="Cam 2 Image", "Image Type"=w18) -> ("New Image"=w17:T1)  [unwired: 2 in, 2 out]
  n3 = Obtain Notifier(name (unnamed)="Robot IP Update", notification data type="IP Addr" ("name (unnamed)")) -> (notifier out=w33:refnum<notifier>)  [unwired: 2 in, 2 out]
  n4 = call "IMAQ Create"("Image Name"="Dashboard Image", "Image Type"=w50) -> ("New Image"=w48:T1, "error out"=w47:errorcluster)  [unwired: 2 in, 1 out]
  n5 = Obtain Notifier(name (unnamed)="Window Mode", notification data type=TRUE) -> (notifier out=w32:refnum<notifier>)  [unwired: 2 in, 2 out]
  n6 = call "624WPIAdjust Dashboard Window.vi"("Width"=i16 1300, "Height"=i16 500, "VI"=w35, "Notifier in"=w32) -> ()  [unwired: 8 in]
  n7 = call "IMAQ Create"("Image Name"="Dashboard Image 2", "Image Type"=w5) -> ("New Image"=w3:T1)  [unwired: 2 in, 2 out]
  n8 = register-events(refnum<vi> refnum) -> (reference out=w39:refnum<event-registration>, error out=w38:errorcluster)  [unwired: 2 in]
  n9 = property class="VI"() -> ("Panel"=w41:refnum<vi>)  [unwired: 2 in, 2 out]
  n10 = while {
    tunnel: w33 -> [w61]
    tunnel: w32 -> [w60]
    stop <- FALSE stop-if-true
    n11 = local read "Vision"() -> (w59:u16)
    n12 = call "624WPI_DashboardGetInfo.vi"("Vision"=w59, "Binding Refnum"=w61, "Window Mode Notifier"=w60, "TCP Cnx"="TCP") -> ("Power and Errors"=w57:T31, "Robot Metrics"=w56:T30, "Status Info"=w55:T29, "Control Info"=w54:T32, "Robot Mode"=w53:T4, "Process?"=w51:bool, "Custom Dashboard Data"=w52:string)  [unwired: 1 in]
    "Robot Mode" <- w53
    n13 = case shown="True" w51 {
      tunnel: w55 -> [_ w134]
      tunnel: w56 -> [_ w129]
      tunnel: w54 -> [_ w128]
      tunnel: w57 -> [_ w133]
      tunnel: w53 -> [_ _]
      tunnel: w52 -> [_ w131]
      frame False {
        (unwired) T6 {"Height"=0.0, "Enc Value"=0.0, "Limit Override"=FALSE, "Mode"=enum."Manual", "High IR"=FALSE, "Motor Out"=0.0, "Ping Detect"=FALSE, "Auto Elevator Indicators"={"Target Out"=0.0, "Storing Trashcan?"=FALSE, "State"=enum."Idle", "In Range"=FALSE, "Store Can Command"=FALSE, "HP Load"=FALSE}, "Master Current"=0.0, "Slave Current"=0.0, "High Current"=FALSE, "Current Tripped"=FALSE, "Top Limit"=FALSE, "Bottom Limit"=FALSE, "Eject Piston"=FALSE, "Stabilizer"=FALSE, "Finger"=FALSE, "Finger Height"=0.0, "Finger Raw"=0.0, "Finger at Bottom"=FALSE} ("Elevator Status Data")
      }
      frame True {
        # "Pressure fancy BG Colors"
        n14 = Unbundle By Name(w133) -> ("Robot IP"=→"Robot IP":string, "Camera Addr"=→"Camera IP":string)
        n15 = Unflatten From String(type=T53 {"Gyro Angle"=0.0, "Autonomous"={"Selected File"="", "Directory"="", "Auton File Index"=0, "Auton File Count"=0, "Auton Command Array"=[]}, "Pressure Transducer V"=0.0, "Pressure"=0.0, "Roller State Indicators"={"Rollers Closed?"=FALSE, "Roller Mode"=enum."Manual", "Auto Roller State"=enum."Grab Tote", "Tote Inside?"=FALSE, "Intake State"=enum."Acquire Tote", "Left Ping Dist"=0.0, "Right Ping Dist"=0.0, "Potentiometer Cluster"={"Left Pot Zero"=0.0, "Right Pot Zero"=0.0, "Left Potentiometer"=0.0, "Right Potentiometer"=0.0, "Left Pot Non Zero"=0.0, "Right Pot Non Zero"=0.0}, "PING Decision"=enum."Acquire Tote", "Left Arm Closed?"=FALSE, "Portrait?"=FALSE, "Right Arm Closed?"=FALSE, "Left Out"=0.0, "Right Out"=0.0, "Left Current"=0.0, "Right Current"=0.0, "Tote Load Complete?"=FALSE, "Untip Complete?"=FALSE, "Untip State"=enum."Idle", "Roller Safety Open"=FALSE}, "Elevator Status Data"={"Height"=0.0, "Enc Value"=0.0, "Limit Override"=FALSE, "Mode"=enum."Manual", "High IR"=FALSE, "Motor Out"=0.0, "Ping Detect"=FALSE, "Auto Elevator Indicators"={"Target Out"=0.0, "Storing Trashcan?"=FALSE, "State"=enum."Idle", "In Range"=FALSE, "Store Can Command"=FALSE, "HP Load"=FALSE}, "Master Current"=0.0, "Slave Current"=0.0, "High Current"=FALSE, "Current Tripped"=FALSE, "Top Limit"=FALSE, "Bottom Limit"=FALSE, "Eject Piston"=FALSE, "Stabilizer"=FALSE, "Finger"=FALSE, "Finger Height"=0.0, "Finger Raw"=0.0, "Finger at Bottom"=FALSE}, "IMU Data"={"Pitch"=0.0, "Roll"=0.0, "Yaw"=0.0, "Data Valid?"=FALSE, "Temp"=0.0, "MOVING"=FALSE, "NAVX_CAL_STATUS"=0, "NAVX_OP_STATUS"=0, "YAW_STABLE"=FALSE, "Accel X"=0.0, "Accel Y"=0.0, "Accel Z"=0.0, "Accel Magnitude"=0.0, "Pitch Rate"=0.0, "Roll Rate"=0.0, "Yaw Rate"=0.0, "NavX Opened?"=FALSE}, "Tote Count"=0, "Have Trashcan"=FALSE, "Encoder Values"={"Left Encoder"={"Distance"=0.0, "Speed"=0.0, "Ticks"=0.0}, "Center Encoder"={"Distance"=0.0, "Speed"=0.0, "Ticks"=0.0}, "Right Encoder"={"Distance"=0.0, "Speed"=0.0, "Ticks"=0.0}}, "Power and Diagnostic Data"={"PDP Data"={"Battery Voltage"=0.0, "Temperature (degrees C)"=0.0, "Internal Battery R (Ohms)"=0.0, "Energy (J)"=0.0, "Power (W)"=0.0, "Total Current (A)"=0.0, "Battery Voltage Fault"=FALSE, "Temperature Fault"=FALSE, "Hardware Fault"=FALSE, "Currents"={"[0]"=0.0, "[1]"=0.0, "[2]"=0.0, "[3]"=0.0, "[4]"=0.0, "[5]"=0.0, "[6]"=0.0, "[7]"=0.0, "[8]"=0.0, "[9]"=0.0, "[10]"=0.0, "[11]"=0.0, "[12]"=0.0, "[13]"=0.0, "[14]"=0.0, "[15]"=0.0}, "Current Faults"={"[0]"=FALSE, "[1]"=FALSE, "[2]"=FALSE, "[3]"=FALSE, "[4]"=FALSE, "[5]"=FALSE, "[6]"=FALSE, "[7]"=FALSE, "[8]"=FALSE, "[9]"=FALSE, "[10]"=FALSE, "[11]"=FALSE, "[12]"=FALSE, "[13]"=FALSE, "[14]"=FALSE, "[15]"=FALSE}}, "PCM Data"={"Compressor Fault"=FALSE, "Solenoid Fault"=FALSE, "Compressor Enabled"=FALSE, "Hardware Fault"=FALSE, "Compressor Current"=0.0}, "roboRIO input voltage (V)"=0.0, "roboRIO input current (A)"=0.0, "3.3V Rail Short"=FALSE, "5 V Rail Short"=FALSE, "6 V Rail Short"=FALSE, "roboRIO Brownout"=FALSE, "Outputs Enabled?"=FALSE}, "Loop Timings"={"Roller Loop"=0, "Elevator Loop"=0, "US Loop"=0, "100ms Loop"=0, "Drivetrain Loop"=0}, "Ultrasonic Data"={"Left Distance"=0.0, "Right Distance"=0.0, "Center Distance"=0.0, "Left Distance Unfilter"=0.0, "Right Distance Unfilter"=0.0, "Center Distance Unfilter"=0.0}, "Zeroing Rollers?"=FALSE, "Drivetrain"={"Y (Throttle)"=0.0, "X (Steer)"=0.0, "Translation X"=0.0, "Center Wheel Down"=FALSE, "Mode"=enum."Manual", "Distance Drive finished?"=FALSE, "Y Target"=0.0, "X Target"=0.0, "Heading Target"=0.0, "Dist Drive Status"={"Y In Range"=FALSE, "X In Range"=FALSE, "Gyro In Range"=FALSE, "Y Dist"=0.0, "X Dist"=0.0, "Gyro"=0.0}, "Step Eject Lockout"=FALSE, "Gyro In Range?"=FALSE, "Yaw Comp Indicators"={"Rate Command"=0.0, "Rate Actual"=0.0, "Steer adjustment"=0.0}}, "Current Auto Command Data"={"Step ID"=0, "Command Type"=0, "Drive X"=0.0, "Drive Y"=0.0, "Heading"=0.0, "Max Exec. Time"=0, "Jump Type"=0, "Jump To"=0, "Jump Condition"=0, "Async Drive?"=0, "Roller Mode"=0, "Roller Align"=0, "Roller Closed?"=0, "Wait Condition"=0, "Elevator Mode"=0, "Elevator Command"=0, "Roller State"=0, "Hold Low?"=0, "Num Totes"=0, "Num Cans"=0.0, "Past Distance"=0.0, "Store Can?"=0.0, "X Speed"=0.0, "Y Speed"=0.0, "Yaw Angle Set"=0.0, "Grab Can"=0.0, "Roller Overide Speed"=0.0, "Force Load?"=0.0, "Set Idle"=0.0, "Eject"=0.0, "Pike Action"=0.0, "Pivot Speed"=0.0, "Height"=0.0}, "Can Grabber"=FALSE, "Pike"={"Motor Out"=0.0, "Current"=0.0, "Limit Switch"=FALSE, "Current Limit"=FALSE, "State"=enum."Going Up", "Command"=enum."Auto Up"}, "Elevator Command"={"Command"=enum."Idle", "Manual Motor Out"=0.0, "Manual Eject Piston"=FALSE, "Mode"=enum."Manual", "Override Limits"=FALSE, "Manual Stabilizer"=FALSE, "Manual Finger"=FALSE, "Store Trashcan?"=FALSE, "Hold Low?"=FALSE, "Idle Mode"=enum."Load Can", "HP Load"=FALSE, "Unstick"=FALSE, "Raw Height Set"=0.0, "Force Store"=FALSE}} ("DB Disp Data"), binary string=w131) -> (value=w114:T53, error out=w130:errorcluster)  [unwired: 3 in, 1 out]
        n16 = call <vilib>:"Clear Errors.vi"("error in (no error)"=w130) -> ()  [unwired: 5 in, 2 out]
        n17 = Unbundle By Name(w114) -> ("Elevator Command"=w72:T49, "Current Auto Command Data"=→"Current Auto Command Data":T14, "Drivetrain"=→"Drivetrain" →"Drivetrain 4":T15, "IMU Data"=w119:T35, "Pressure"=w106:dbl, "Pressure Transducer V"=→"Transducer Voltage":dbl, "Gyro Angle"=→"Gyro":dbl, "Power and Diagnostic Data"=→"Power and Diagnostic Data":T26, "Autonomous"=w115:T54, "Roller State Indicators"=w88:T41, "Encoder Values"=→"Encoder Values":T38, "Elevator Status Data"=w81:T6, "Zeroing Rollers?"=→"Zeroing Rollers?":bool)  [unwired: 1 out]
        "Pressure" <- w106
        "Roller State Indicators" <- w88
        "Pressure 2" <- w106
        "IMU Data" <- w119
        "Elevator Status Data 2" <- w81
        "Elevator Status Data 3" <- w81
        "Elevator Command" <- w72
        n18 = Unbundle By Name(w114) -> ("Have Trashcan"=→"Trashcan? 2" →"Trashcan?":bool, "Loop Timings"=→"Loop Timings":T33, "Ultrasonic Data"=→"Ultrasonic Data" →"Ultrasonic Data 2" →"Ultrasonic Data 3":T5)  [unwired: 1 out]
        n19 = Unbundle By Name(w72) -> ("Command"=→"Elev Command":T12, "Idle Mode"=→"Idle Mode":T13)
        n20 = Unbundle By Name(w115) -> ("Selected File"=→"Current File" →"Auton File":string, "Directory"=→"Directory":string, "Auton File Index"=→"File Index":i32, "Auton File Count"=→"Auton File Count":i32)
        n21 = Unbundle By Name(w119) -> ("NAVX_CAL_STATUS"=→"NAVX_CAL_STATUS":T3, "Roll"=→"Roll":sgl, "Pitch"=→"Pitch":sgl, "Yaw"=→"IMU Gyro":sgl)
        n22 = local read "Elevator"() -> (w68:T47)
        n23 = Unbundle By Name(w81) -> ("Mode"=w94:T7, "Finger"=→"Finger":bool, "Stabilizer"=→"Stabilizer":bool, "Eject Piston"=→"Eject":bool, "High IR"=w65:bool, "Finger Height"=w69:dbl)
        n24 = Unbundle By Name(w68) -> ("Finger max"=w67:dbl)
        n25 = Greater Or Equal?(x=w69, y=w67) -> (x >= y?=w66:bool)
        n26 = Unbundle By Name(w88) -> ("Roller Mode"=w87:T11)
        n27 = Or(x=w65, y=w66) -> (x .or. y?=→"Elev Limit":bool)
        n28 = Unbundle By Name(w88) -> ("Rollers Closed?"=w110:bool, "Roller Mode"=w108:T11, "Left Out"=w77:sgl, "Right Out"=w76:sgl, "Left Current"=w75:sgl, "Right Current"=w74:sgl)
        n29 = case shown="\"Auto\"" w94 {
          tunnel: [u32 16711680 u32 16772394 u32 6618880] -> w97
          tunnel: ["MANUAL" "SAFE" "AUTO"] -> w89
          frame "Manual", Default {
          }
          frame "Safe" {
          }
          frame "Auto" {
          }
        }
        n30 = case shown="\"Auto\"" w87 {
          tunnel: [u32 16711680 u32 16772394 u32 6618880] -> w92
          tunnel: ["MANUAL" "SAFE" "AUTO"] -> w90
          frame "Manual", Default {
          }
          frame "Safe" {
          }
          frame "Auto" {
          }
        }
        n31 = Greater Or Equal?(x=w106, y=70.0) -> (x >= y?=w104:bool)
        n32 = Greater Or Equal?(x=w106, y=50.0) -> (x >= y?=w101:bool)
        n33 = Select(t=u32 16772394, s=w101, f=u32 16711680) -> (s? t:f=w102:u32)
        n34 = Bundle By Name(cluster=T10 {"Rollers Closed?"=FALSE, "Roller Mode"=enum."Manual", "Left Out"=0.0, "Right Out"=0.0, "L Current"=1.0, "R Current"=1.0} ("Roller Indicators Thin"), "Rollers Closed?"=w110, "Roller Mode"=w108, "Left Out"=w77, "Right Out"=w76, "L Current"=w75, "R Current"=w74) -> (→"Roller Indicators Thin":T10)
        n35 = Select(t=u32 6618880, s=w104, f=w102) -> (s? t:f=w98:u32)
        n36 = Bundle(w97, w97) -> (w96:cluster{u32, u32})  [unwired: 1 in]
        n37 = Bundle(w92, w92) -> (w93:cluster{u32, u32})  [unwired: 1 in]
        n38 = property on="Pressure" class="DigNum (strict)"("NumText.BGColor"=w98) -> ()  [unwired: 2 in, 2 out]
        n39 = property on="Pressure 2" class="DigNum (strict)"("NumText.BGColor"=w98) -> ()  [unwired: 2 in, 2 out]
        n40 = Build Array(w96, w96) -> (w95:cluster{u32, u32}[])
        n41 = Build Array(w93, w93) -> (w91:cluster{u32, u32}[])
        n42 = property on="Elevator Mode" class="Bool (strict)"("BoolText.Text"=w89, "Colors [4]"=w95) -> ()  [unwired: 2 in, 2 out]
        n43 = property on="Roller Mode" class="Bool (strict)"("BoolText.Text"=w90, "Colors [4]"=w91) -> ()  [unwired: 2 in, 2 out]
        "Status Info" <- w134
        "Robot Metrics" <- w129
        "DS TCP" <- w133
        "Control Info" <- w128
      }
    }
  }
  n44 = vi-ref "Playback Controls.vi"() -> (w40:refnum<vi>)
  n45 = call "Initialize Camera and CheckList.vi"() -> ("Cluster"=w28:cluster{"value":i32, "value":i32, "index":i32}, "Array"=w27:cluster{string[]}[], "File Refnum"=w26:T58)  [unwired: 9 in]
  n46 = property class="Pnl"(reference=w41) -> ("Panes[]"=w42:refnum<vi>[])  [unwired: 1 in, 2 out]
  n47 = while {
    stop <- FALSE stop-if-true
    # "Send control parameters to robot 4x per second on UDP port 5801"
    n48 = Wait (ms)(milliseconds to wait=u32 250) -> ()  [unwired: 1 out]
    n49 = Bundle By Name(cluster=T59 {"Cam Exposure"=0.0, "Go to angle"=0.0, "Steer PID Gains"={"proportional gain (Kc)"=1.0, "integral time (Ti, min)"=0.01, "derivative time (Td, min)"=0.0}, "Steer PID output Range"={"output high"=1.0, "output low"=-1.0}, "Pressure m \nValue"=0.0, "Pressure b \nValue"=0.0, "Roller Command Cluster "={"Intake Speed"=0.0, "Turn In Speed"=0.0, "Unload Speed"=0.0, "Turn Out Speed"=0.0, "Ping Align Tolerance"=1000.0, "Tote Range Threshold"=0.0, "Right Pot 0"=0.0, "Pot Threshold"=0.0, "Left Pot 0"=0.0, "Right Pot Scale"=0.0, "Left Pot Scale"=0.0, "Min Elevator Height"=0.0, "Eject Time"=0.0, "Eject US Threshold"=0.0, "Anti-Twitch Time"=0, "Ping Caring Threshold"=0.0, "Pot Diff Threshold"=0.0, "Pinch Sustain"=0, "Absorb Give Up Threshold"=0.0, "Untip In Threshold"=0.0, "Untip Grab Range"=0.0, "Ultrasonic Hold Time"=0, "Landscape Absorb Time"=0, "Pot Use Wait Time"=0, "Can Turn Stop Range"=0.0, "HP Load Speed"=0.0, "Stick Multiplier"=0.0, "Coop Eject Speed"=0.0}, "Elevator"={"PID Output Range"={"output high"=100.0, "output low"=-100.0}, "PID gains"={"proportional gain (Kc)"=1.0, "integral time (Ti, min)"=0.01, "derivative time (Td, min)"=0.0}, "Height Tolerance"=0.0, " Encoder Constant"=0.0, "Eject Time"=0.0, "Zeroing Speed"=0.0, "Presets"={"Pickup 2 w/ Tote"=0.0, "Pickup 2 w/ Trashcan"=0.0, "Pickup 3 w/ Tote"=0.0, "Pickup 3 w/ Trashcan"=0.0, "Bottom"=0.0, "Pickup 1 w/ Tote"=0.0, "Pickup Trashcan"=0.0, "Pickup 1 w/ Trashcan"=0.0, "Eject"=0.0, "Hold Low"=0.0, "Step add height"=0.0, "Untip Lift"=0.0, "Drop Stack"=0.0, "HP Load Hold"=0.0, "HP Load Drop"=0.0, "HP Load Hold Can"=0.0, "Store can max"=0.0, "HP Drag Score"=0.0, "HP Drag Finish"=0.0, "Finger trashcan avoid"=0.0, "Full"=0.0}, "Ping Detect Threshold"=0.0, "Trashcan Detect Threshold"=0.0, "Zero Filter Time"=0.0, "Stabilizer Open Time"=0.0, "Zero Creep Speed"=0.0, "Max Current"=0.0, "Current Trip Time"=0.0, "Abort Pitch"=0.0, "Finger m"=0.0, "Finger b"=0.0, "Finger max "=0.0, "Finger Stabilizer"=0.0, "Finger Store"=0.0, "Finger Stop Store"=0.0, "Stabilizer Close Time"=0.0, "Finger min"=0.0, "Unstick gain"=0.0, "Full Detect Max"=0.0}, "Encoder Control"={"Left Tick Constant"=1.0, "Right Tick Constant"=0.0, "Center Tick Constant"=0.0, "Reset?"=FALSE, "Y Dist"={"PID gains"={"proportional gain (Kc)"=1.0, "integral time (Ti, min)"=0.0, "derivative time (Td, min)"=0.0}}, "X Dist"={"PID gains"={"proportional gain (Kc)"=1.0, "integral time (Ti, min)"=0.0, "derivative time (Td, min)"=0.0}}, "Y Stop Thresh"=0.0, "Y Stop Speed"=0.0, "X Stop Thresh"=0.0, "X Stop Speed"=0.0}, "Auton Settings"={"Drive Dist Window Size"=0.0}, "Drivetrain Settings"={"Gyro Tolerance"=0.0, "Strafe Correct max steer"=0.4, "Strafe Timer Wait"=250.0, "Throttle Ramp (ms)"=0.0, "Strafe Ramp (ms)"=0.0, "Angular rate compensation"=FALSE, "Throttle to Rate Scale"=0.0, "Rate compensation gain"=0.0, "Creep Steer"=0.0, "Creep Throttle"=0.0}, "Lance"={"Down Speed"=0.0, "Up Speed"=0.0, "Max Down Time"=0.0, "Max Up Time"=0.0, "Current Limit"=0.0}} ("DB Control Data"), "Cam Exposure"="Cam Exposure", "Go to angle"="Go to angle", "Steer PID Gains"="Yaw PID Gains", "Steer PID output Range"="Yaw PID Output Range", "Pressure m \nValue"="Pressure m Value", "Pressure b \nValue"="Pressure b Value", "Roller Command Cluster"="Roller Settings", "Elevator"="Elevator", "Encoder Control"="Encoder Control", "Drivetrain Settings"="Drivetrain Settings") -> (w148:T59)
    n50 = Flatten To String(anything=w148) -> (data string=w147:string)  [unwired: 3 in, 2 out]
    n51 = local read "Robot IP"() -> (w160:string)
    n52 = call "DumbDash Send.vi"("Robot IP"=w160, "data string"=w147) -> ()  [unwired: 10 in]
  }
  n53 = property on="Camera Settings" class="Clust (strict)"("Val(Sgnl)"=w28) -> ()  [unwired: 2 in, 2 out]
  n54 = Index Array(array=w42) -> (element=w25:refnum<vi>)  [unwired: 1 in]
  n55 = while {
    tunnel: w27 -> [w169]
    shift-right: [w168] -> _
    shift-left: w26 -> [w167]
    tunnel: [w166] -> _
    tunnel: w40 -> [w165]
    tunnel: w39 -> [w164]
    tunnel: w38 -> [_]
    tunnel: w35 -> [w163]
    i -> [w166]
    stop <- FALSE stop-if-true
    n56 = event shown="[2] \"Rec Mode\": Value Change" {
      selector: w164 -> [_ _ _ _ _ _]
      dyn-events: [_ _ w213 _ _ _] -> _
      timeout: _ -> [_ _ _ _ _ _]
      tunnel: w169 -> [w173 w203 _ _ _ _]
      tunnel: [w172 w196 w215 w229 w230 w240] -> w168
      tunnel: w167 -> [w171 w196 w215 w229 w230 w240]
      tunnel: w165 -> [_ _ w216 _ w233 _]
      tunnel: w163 -> [_ _ w211 _ _ _]
      event "DB Camera Config": Value Change {
        # "Show or hide the cluster of controls, store in ini file"
        n57 = event-data() -> ("NewVal"=w174:bool)  [unwired: 1 in]
        n58 = case shown="False" w174 {
          tunnel: w173 -> [w183 _]
          tunnel: [w176 w194] -> w172
          tunnel: w171 -> [w175 w194]
          frame False {
            w190 = "Camera"
            w193 = FALSE ("Visible")
            n59 = local read "Camera Settings"() -> (w182:T19)
            n60 = Index Array(array=w183) -> (element=w186:cluster{string[]})  [unwired: 1 in]
            n61 = Unbundle(w182) -> ("Frame Rate"=w181:i32, "Compression"=w180:i32, "Size"=w184:u16)
            n62 = Unbundle(w186) -> (w185:string[])
            n63 = Index Array(array=w185, index=w184) -> (element=w179:string)
            n64 = call-poly <vilib>:"Write Key.vi"("section"=w190, "value"=w179, "key"="Size", "refnum"=w175) -> ("refnum out"=w192:T58)  [unwired: 2 in, 5 out]
            n65 = call-poly <vilib>:"Write Key.vi"("section"=w190, "value"=w181, "key"="FrameRate", "refnum"=w192) -> ("refnum out"=w191:T58)  [unwired: 1 in, 6 out]
            n66 = property on="Camera Settings" class="Clust (strict)"("Visible"=w193) -> ()  [unwired: 2 in, 2 out]
            n67 = local write "DB Camera Config"(w193) -> ()
            n68 = call-poly <vilib>:"Write Key.vi"("section"=w190, "value"=w180, "key"="Compression", "refnum"=w191) -> ("refnum out"=w177:T58)  [unwired: 1 in, 6 out]
            n69 = call <vilib>:"Close Config Data.vi"("refnum"=w177) -> ("file path"=w178:path)  [unwired: 2 in, 8 out]
            n70 = call <vilib>:"Open Config Data.vi"("configuration file path"=w178) -> ("refnum"=w176:T58)  [unwired: 8 in, 2 out]
          }
          frame True {
            n71 = property on="Camera Settings" class="Clust (strict)"("Visible"=TRUE) -> ()  [unwired: 2 in, 2 out]
          }
        }
      }
      event "Camera Settings": Value Change {
        # "Update summary string when any elements of DB camera change"
        n72 = event-data() -> ("NewVal"=w207:T19)  [unwired: 1 in]
        n73 = Index Array(array=w203) -> (element=w202:cluster{string[]})  [unwired: 1 in]
        n74 = Unbundle(w207) -> ("Frame Rate"=w198:i32, "Compression"=w197:i32, "Size"=w200:u16)
        n75 = Unbundle(w202) -> (w201:string[])
        n76 = Index Array(array=w201, index=w200) -> (element=w199:string)
        n77 = Format Into String(format string="%s   %dfps   %d%%", w199, w198, w197) -> (resulting string=w204:string)  [unwired: 2 in, 1 out]
        n78 = Build Array(w204) -> (w205:string[])
        n79 = property on="DB Camera Config" class="Bool (strict)"("Strings [4]"=w205) -> ()  [unwired: 2 in, 2 out]
      }
      event "Rec Mode": Value Change {
        # "Update globals for recording mode and path to read log from.\nClear when logging and let NetworkTables set path for vision to\nuse."
        n80 = event-data() -> ("NewVal"=w217:enum32{"Stop", "Record", "Playback"})  [unwired: 1 in]
        n81 = global write "WPI_DashboardLogging Global.vi" "Logging Filename"(path "") -> ()
        n82 = case shown="\"Playback\"" w217 {
          tunnel: w216 -> [_ w219 w223]
          tunnel: [_ _ w227] -> w213
          tunnel: [_ _ w226] -> _
          tunnel: w211 -> [_ _ w221]
          tunnel: cluster{i32, i32} {-250, 170} -> [_ _ w220]
          tunnel: [_ _ T61 {"Image Size"=TRUE, "Image Type"=TRUE, "Pixel Value"=TRUE, "ROI Information"=TRUE, "Zoom Factor"=FALSE} ("Image Information Shown:All Elements")] -> w209
          tunnel: [_ _ TRUE ("Zoom Factor")] -> w208
          frame Default {
          }
          frame "Stop", "Record" {
            # "Place Window too"
            n83 = invoke class="VI" method="FP.Close"(reference=w219) -> (reference out=w218:refnum<vi>)  [unwired: 2 in, 2 out]
            n84 = invoke class="VI" method="Abort VI"(reference=w218) -> ()  [unwired: 2 in, 3 out]
          }
          frame "Playback" {
            n85 = call "Open Playback Panel.vi"("Offset"=w220, "DB VI Ref"=w221, "Playback in"=w223) -> ("Playback out"=w222:refnum<vi>)  [unwired: 8 in]
            n86 = register-events(w222) -> (reference out=w227:refnum<event-registration>, error out=w226:errorcluster)  [unwired: 2 in]
          }
        }
        n87 = global write "WPI_DashboardLogging Global.vi" "Recording"(w217) -> ()
        n88 = property on="Axis Display" class="ImageControl"("Image Information Shown"=w209, "Image Information Visible"=w208) -> ()  [unwired: 2 in, 2 out]
        n89 = call <vilib>:"WPI_DashboardNT Log FieldName Cache.vi"("Operation"=enum16{"Lookup/Add", "Index", "Clear"}."Clear") -> ()  [unwired: 8 in, 3 out]
      }
      event Panel Close {
        w228 = enum32{"Stop", "Record", "Playback"}."Stop" ("Rec Mode")
        # "Playback window has been closed, abort"
        n90 = event-data() -> ()  [unwired: 1 in, 4 out]
        n91 = local write "Rec Mode"(w228) -> ()
        n92 = global write "WPI_DashboardLogging Global.vi" "Recording"(w228) -> ()
      }
      event Panel Close {
        # "Abort playback window and ourself"
        n93 = event-data() -> ()  [unwired: 1 in, 4 out]
        n94 = invoke class="VI" method="FP.Close"(reference=w233) -> (reference out=w232:refnum<vi>)  [unwired: 2 in, 2 out]
        n95 = invoke class="VI" method="Abort VI"(reference=w232) -> (error out=w231:errorcluster)  [unwired: 2 in, 2 out]
        n96 = invoke class="VI" method="Abort VI"(error in=w231) -> ()  [unwired: 2 in, 3 out]
      }
      event "Vision": Value Change {
        # "Enable/Disable Compression slider.\nHW USB is hard-coded into the camera"
        n97 = event-data() -> ("NewVal"=w239:u16)  [unwired: 1 in]
        n98 = Equal?(x=w239, y=u32 2 ("milliseconds to wait")) -> (x = y?=w237:bool)
        n99 = Select(t=T62."Disabled and Grayed Out" ("Disabled"), s=w237, f=T62."Enabled" ("Disabled")) -> (s? t:f=w234:T62)
        n100 = property on="Compression" class="Slide (strict)"("DisabledEnum"=w234) -> ()  [unwired: 2 in, 2 out]
      }
    }
  }
  n101 = while {
    tunnel: w25 -> [w242]
    i -> [w245]
    stop <- FALSE stop-if-true
    n102 = Wait (ms)(milliseconds to wait=u32 100) -> ()  [unwired: 1 out]
    n103 = case shown="\"Playback\"" "Rec Mode" {
      tunnel: w245 -> [_ _ w260]
      tunnel: [u32 1973790 ("Base Color") u32 11141120 ("Target Color") w252] -> w241
      frame "Stop", Default {
        # "Reset the color, extra updates don't cost much"
      }
      frame "Record" {
      }
      frame "Playback" {
        # "Playback"
        n104 = Quotient & Remainder(x=w260, y=u32 50 ("milliseconds to wait")) -> (x-y*floor(x/y)=w256:u32)  [unwired: 1 out]
        n105 = Divide(x=w256, y=u32 50 ("milliseconds to wait")) -> (x/y=w253:dbl)
        n106 = Multiply(x=6.283185307179586, y=w253) -> (x*y=w258:dbl)
        n107 = Sine(x=w258) -> (sin(x)=w257:dbl)
        n108 = Absolute Value(x=w257) -> (abs(x)=w251:dbl)
        n109 = call "Interpolate RGB Color.vi"("Proportion"=w251, "Target Color"=u32 30976, "Base Color"=u32 2829099) -> ("Result Color"=w252:u32)  [unwired: 8 in]
      }
    }
    n110 = property class="Pane"(reference=w242, "PaneColor"=w241) -> ()  [unwired: 1 in, 2 out]
  }
  n111 = property class="Pane"(reference=w25, "Origin"=T52 {"Horizontal"=-1561, "Vertical"=-62}) -> ()  [unwired: 1 in, 2 out]
  n112 = while {
    tunnel: u16 1741 ("timeout ms (25000)") -> [w264]
    stop <- FALSE stop-if-true
    n113 = TCP Create Listener(10:w264) -> (0:w261:errorcluster, 3:w263:refnum<k5>)  [unwired: 4 in, 1 out]
    n114 = case shown="No Error" w261 {
      tunnel: w263 -> [w265 _]
      frame No Error {
        # "Loop 7. Wait for DS connections"
        n115 = while {
          tunnel: w265 -> [w268]
          stop <- FALSE stop-if-true
          n116 = TCP Wait On Listener(11:w268) -> (0:w266:errorcluster, 4:w267:refnum<k5>)  [unwired: 3 in, 3 out]
          n117 = local write "TCP"(w267) -> ()
          n118 = case shown="Error" w266 {
            frame No Error {
            }
            frame Error {
              n119 = Wait (ms)(milliseconds to wait=u32 100) -> ()  [unwired: 1 out]
            }
          }
        }
      }
      frame Error {
      }
    }
  }
  n120 = property on="Camera Settings" class="Clust (strict)"("Visible"=w34) -> ()  [unwired: 2 in, 2 out]
  n121 = local write "DB Camera Config"(w34) -> ()
  n122 = call <vilib>:"Intialize Keyboard.vi"() -> ("device ID"=w7:refnum<k1>)  [unwired: 10 in, 1 out]
  n123 = while {
    tunnel: w7 -> [w273]
    stop <- FALSE stop-if-true
    # "(Keyboard: UDP 5803)"
    # "Send the keyboard to the robot every 50 ms"
    n124 = call-poly <vilib>:"Acquire Input Data.vi"("device ID"=w273) -> ("keys pressed"=w272:T63)  [unwired: 16 in, 2 out]
    n125 = local read "Robot IP"() -> (w271:string)
    n126 = call "Send Keyboard Data.vi"("Robot IP"=w271, "keys pressed"=w272) -> ()  [unwired: 10 in]
    n127 = Wait (ms)(milliseconds to wait=u32 50) -> ()  [unwired: 1 out]
  }
  n128 = global write "WPI_DashboardLogging Global.vi" "Recording"(w36) -> ()
  n129 = local write "Rec Mode"(w36) -> ()
  n130 = Generate Occurrence() -> (w6:refnum<k4>)
  n131 = while {
    tunnel: w48 -> [w283]
    tunnel: w47 -> [_]
    tunnel: w6 -> [w277]
    tunnel: w3 -> [w276]
    stop <- FALSE stop-if-true
    # "Axis cam"
    n132 = case shown="False" "Use File" {
      tunnel: w283 -> [w294 w302]
      tunnel: [w293 w301] -> w282
      tunnel: [w292 w295] -> w281
      tunnel: [w291 62.4 ("FPS")] -> w280
      tunnel: [w290 6.24 ("Bandwidth (Mbps)")] -> w279
      frame False {
        # "Optionally read the DB image,\nlog, or retrieve images from a\nlogged match"
        n133 = local read "Rec Mode"() -> (w288:enum32{"Stop", "Record", "Playback"})
        n134 = call "624WPI_CameraRead MJPG for Dashboard.vi"("Camera Settings"="Camera Settings", "USB Cam TCP Port"=u16 5800, "Rec Mode"=w288, "Camera IP"="axis-camera.local", "Camera Mode"="Camera Mode", "Refnum in"=w294) -> ("Active"=w292:bool, "Refnum out"=w293:T1, "FPS"=w291:dbl, "Bandwidth (Mbps)"=w290:dbl)  [unwired: 2 in]
      }
      frame True {
        n135 = call "IMAQ ReadFile"("File Path"="File Path", "Image"=w302) -> ("error out"=w297:errorcluster, "Image Out"=w301:T1)  [unwired: 5 in, 3 out]
        n136 = Unbundle By Name(w297) -> ("status"=w296:bool)
        n137 = Not(x=w296) -> (.not. x?=w295:bool)
      }
    }
    n138 = case shown="True" w281 {
      tunnel: w282 -> [_ w313]
      tunnel: w279 -> [_ w312]
      tunnel: w280 -> [_ w311]
      tunnel: w277 -> [_ w310]
      tunnel: w276 -> [_ w304]
      frame False {
        # "Sleep for 500ms"
        n139 = Wait Until Next ms Multiple(millisecond multiple=u32 500) -> ()  [unwired: 1 out]
      }
      frame True {
        # "Update Mbps LED"
        n140 = call "IMAQ Clear Overlay"("Image"=w313) -> ("error out"=w317:errorcluster, "Image Out"=w307:T1)  [unwired: 2 in, 7 out]
        n141 = case shown="4, 5" w312 {
          tunnel: [u32 6618880 ("Color Box") u32 16776722 ("Color Box") u32 16716800 ("Color Box")] -> w314
          frame Default {
          }
          frame 4, 5 {
          }
          frame 6.. {
          }
        }
        n142 = Unbundle By Name(w317) -> ("status"=w318:bool)
        n143 = Bundle("Color Box"=w314, "Color Box"=w314) -> (w316:cluster{"Color Box":u32, "Color Box":u32})  [unwired: 1 out]
        n144 = property on="Image Message" class="Str"("Visible"=w318) -> ()  [unwired: 2 in, 2 out]
        n145 = Build Array(w316) -> (w315:cluster{"Color Box":u32, "Color Box":u32}[])
        n146 = disable-structure shown="Enabled" {
          disable-tunnel: [w327 _] -> _
          disable-tunnel: [w326 _] -> _
          disable-tunnel: [w323 w332] -> w309
          disable-tunnel: w307 -> [w320 w334]
          disable-tunnel: [w319 w331] -> w305
          disable-tunnel: w304 -> [_ w330]
          frame Disabled {
            n147 = call "624 Detect Retroreflective Vision Totes.vi"("Limit %"="Min target size %", "Filter Settings"="Filter Settings", "Ring Light Color"="Ring Light Color", "Image Src"=w320, "Camera FOV width"="Camera FOV width") -> ("Detected totes"=w327:T24[], "Masked"=w324:T1, "Processed Img"=w319:T1)  [unwired: 4 in]
            "Detected totes" <- w327
            n148 = local read "Robot IP"() -> (w326:string)
            n149 = Select(t=w324, s="Mask View", f=w319) -> (s? t:f=w323:T1)
          }
          frame Enabled {
            n150 = call "Draw Feeder Overlay.vi"("Rectangle"="Rectangle", "Refnum in"=w334) -> ("Refnum out"=w332:T1)  [unwired: 9 in]
            n151 = call "IMAQ Copy"("Image Dst"=w330, "Image Src"=w332) -> ("Image Dst Out"=w331:T1)  [unwired: 4 in, 1 out]
          }
        }
        "Axis Display" <- w309
        "Axis Cam" <- w305
        n152 = property on="Mbps 2" class="Bool (strict)"("Colors [4]"=w315) -> ()  [unwired: 2 in, 2 out]
        n153 = control-ref of="Axis Display"() -> (w308:refnum<vi>)
        n154 = control-ref of="Ring Light Color"() -> (w306:refnum<vi>)
        n155 = call "Calibration Helper.vi"("Color Display"=w306, "Image"=w307, "Image Ctl Refnum"=w308) -> ()  [unwired: 8 in, 1 out]
        n156 = Set Occurrence(w310) -> ()
        "Mbps" <- w312
        "fps" <- w311
      }
    }
  }
  n157 = while {
    tunnel: w17 -> [w349]
    tunnel: w6 -> [w338]
    stop <- FALSE stop-if-true
    # "USB Cam here"
    n158 = local read "Camera IP"() -> (w348:string)
    n159 = local read "Rec Mode"() -> (w346:enum32{"Stop", "Record", "Playback"})
    n160 = call "624WPI_CameraRead MJPG for Dashboard.vi"("Camera Settings"="Camera Settings 2", "USB Cam TCP Port"=u16 1180, "Rec Mode"=w346, "Camera IP"=w348, "Camera Mode"="Vision", "Refnum in"=w349) -> ("Active"=w344:bool, "Refnum out"=w343:T1, "FPS"=w340:dbl, "Bandwidth (Mbps)"=w342:dbl)  [unwired: 2 in]
    n161 = case shown="True" w344 {
      tunnel: w343 -> [_ w352]
      tunnel: w342 -> [_ w354]
      tunnel: w340 -> [_ w353]
      tunnel: w338 -> [_ w351]
      frame False {
        n162 = Wait Until Next ms Multiple(millisecond multiple=u32 500) -> ()  [unwired: 1 out]
      }
      frame True {
        n163 = Set Occurrence(w351) -> ()
        "USB Cam" <- w352
        "Mbps 2" <- w354
        "fps 2" <- w353
      }
    }
  }
  n164 = vi-ref "Image Display.vi"() -> (w9:refnum<vi>)
  n165 = while {
    tunnel: w6 -> [w358]
    stop <- FALSE stop-if-true
    n166 = local read "Mbps"() -> (w357:dbl)
    n167 = local read "Mbps 2"() -> (w356:dbl)
    n168 = Wait on Occurrence(2:w358) -> ()  [unwired: 2 in, 1 out]
    n169 = Add(x=w357, y=w356) -> (x+y=→"Total mbps":dbl)
    n170 = local read "USB Cam"() -> (w360:T1)
    n171 = local read "Axis Cam"() -> (w359:T1)
    n172 = call "Image Display.vi"("Img In 2"=w360, "Img In"=w359) -> ()  [unwired: 10 in]
  }
  n173 = control-ref of="Dashboard Tab"() -> (w13:refnum<vi>)
  n174 = invoke class="VI" method="FP.Open"(reference=w9, "Activate"=TRUE ("Activate?"), "State"=T51."Standard") -> (reference out=w12:refnum<vi>)  [unwired: 2 in, 4 out]
  n175 = call "DumbDash Load Controls.vi"("TabControl in"=w13) -> ("Array"=w16:T64[])  [unwired: 10 in]
  n176 = property class="VI"(reference=w12, "Front Panel.ShowMenuBar"=w8, "TB.Visible"=w8, "Front Panel.Resizeable"=w8) -> ()  [unwired: 1 in, 2 out]
  n177 = call <vilib>:"Read PNG File.vi"("path to PNG file"=path "tote_stack_pics/gray_tote.png" ("path to JPEG file")) -> ("image data"=w22:T66)  [unwired: 8 in, 2 out]
  n178 = control-ref of="DumbDash Message"() -> (w15:refnum<vi>)
  n179 = while {
    tunnel: w16 -> [w373]
    tunnel: w15 -> [w372]
    stop <- FALSE stop-if-true
    n180 = local read "Robot IP"() -> (w366:string)
    n181 = local read "Camera IP"() -> (w370:string)
    n182 = local read "Robot IP"() -> (w371:string)
    n183 = Equal?(x=w366, y="0.0.0.0") -> (x = y?=w364:bool)
    n184 = Empty String/Path?(string/path=w370) -> (empty?=w368:bool)
    n185 = Empty String/Path?(string/path=w371) -> (empty?=w369:bool)
    n186 = case shown="True" "Save" {
      tunnel: w373 -> [_ w389]
      tunnel: w372 -> [_ w388]
      frame False {
      }
      frame True {
        n187 = flat-sequence {
          tunnel: w389 -> [w391]
          tunnel: w388 -> [w390]
          frame #0 {
            n188 = call "DumbDash Save Values.vi"("Message Box"=w390, "Controls In"=w391) -> ()  [unwired: 10 in]
          }
          frame #1 {
            n189 = local write "Save"(FALSE ("Save")) -> ()
          }
        }
      }
    }
    n190 = case shown="True" "Load" {
      tunnel: w373 -> [_ w384]
      tunnel: w372 -> [_ w383]
      frame False {
      }
      frame True {
        n191 = flat-sequence {
          tunnel: w384 -> [w386]
          tunnel: w383 -> [w385]
          frame #0 {
            n192 = call "DumbDash Load Values.vi"("Message Box"=w385, "Controls In"=w386) -> ()  [unwired: 10 in]
          }
          frame #1 {
            n193 = local write "Load"(FALSE ("Load")) -> ()
          }
        }
      }
    }
    n194 = Compound Arithmetic op=OR(w364, w369, w368) -> (w367:bool)
    n195 = case shown="True" w367 {
      frame False {
        n196 = property on="DumbDash Message" class="Str"("Blinking"=FALSE) -> ()  [unwired: 2 in, 2 out]
      }
      frame True {
        n197 = disable-structure shown="Disabled" {
          frame Disabled {
            w382 = u32 16711680
            n198 = property on="DumbDash Message" class="Str"("Blinking"=TRUE, "Text.BGColor"=w382, "Text.BG Color"=w382) -> ()  [unwired: 2 in, 2 out]
            "DumbDash Message" <- "Restart the Driver Station!! Bad IP" ("DumbDash Message")
          }
          frame Enabled {
          }
        }
      }
    }
    n199 = disable-structure shown="RUN_TIME_ENGINE==True" {
      disable-tunnel: "stop" -> [w377 w378]
      frame condition #0 {
        # "Close the build DB"
        n200 = Quit LabVIEW(quit? (T)=w377) -> ()
      }
      frame condition #1 (active) {
        n201 = Stop(stop? (T)=w378) -> ()
      }
    }
    n202 = Wait (ms)(milliseconds to wait=u32 250) -> ()  [unwired: 1 out]
  }
  n203 = while {
    stop <- FALSE stop-if-true
    # "Clear the background of the message\nbox after a while"
    n204 = event shown="[0] \"DumbDash Message\": Value Change" {
      selector: _ -> [_]
      dyn-events: _ -> [_]
      timeout: _ -> [_]
      event "DumbDash Message": Value Change {
        n205 = event-data() -> ()  [unwired: 1 in, 3 out]
        n206 = flat-sequence {
          frame #0 {
            n207 = Wait (ms)(milliseconds to wait=u32 3000) -> ()  [unwired: 1 out]
          }
          frame #1 {
            w396 = u32 3552822
            n208 = property on="DumbDash Message" class="Str"("Text.BGColor"=w396, "Text.BG Color"=w396, "Blinking"=FALSE) -> ()  [unwired: 2 in, 2 out]
          }
        }
      }
    }
  }
  n209 = while {
    shift-right: [w404] -> _
    shift-left: 0 -> [w405]
    shift-right: [w399] -> _
    shift-left: _ -> [w400]
    tunnel: path "Dashboard Code/memes/Oh_Baby_A_Triple.wav" ("path") -> [w397]
    stop <- FALSE stop-if-true
    n210 = local read "Pressure"() -> (w402:dbl)
    n211 = Less?(x=w402, y=95.0) -> (x < y?=w403:bool)
    n212 = case shown="True" w403 {
      tunnel: w405 -> [_ w433]
      tunnel: [0 w423] -> w404
      tunnel: [picture data[5B] ("new picture") w428] -> w399
      tunnel: w400 -> [_ _]
      frame False {
      }
      frame True {
        n213 = property on="2D Picture" class="Pict"() -> ("Draw Area Size"=w421:T67)  [unwired: 2 in, 2 out]
        n214 = Number To Decimal String(number=w433) -> (decimal integer string=w431:string)  [unwired: 1 in]
        n215 = Unbundle By Name(w421) -> ("Width"=w416:u32, "Height"=w419:u32)
        n216 = Concatenate Strings("pump_tire\\frame_", w431, "_delay-0.1s.png") -> (w429:string)
        n217 = Increment(x=w433) -> (x+1=w425:i32)
        n218 = String To Path(string=w429) -> (path=w422:path)
        n219 = Less Or Equal?(x=w425, y=7) -> (x <= y?=w426:bool)
        n220 = call <vilib>:"Read PNG File.vi"("path to PNG file"=w422) -> ("image data"=w420:T66)  [unwired: 8 in, 2 out]
        n221 = Unbundle By Name(w420) -> ("Rectangle.right"=w417:i16, "Rectangle.bottom"=w418:i16)
        n222 = Divide(x=w416, y=w417) -> (x/y=w414:dbl)
        n223 = Divide(x=w419, y=w418) -> (x/y=w415:dbl)
        n224 = Max & Min(x=w414, y=w415) -> (min(x,y)=w413:dbl)  [unwired: 1 out]
        n225 = Select(t=w425, s=w426, f=0) -> (s? t:f=w423:i32)
        n226 = call <vilib>:"Draw Flattened Pixmap.vi"("image data"=w420) -> ("new picture"=w428:picture)  [unwired: 8 in]
        n227 = property on="2D Picture" class="Pict"("ZoomFactor"=w413) -> ()  [unwired: 2 in, 2 out]
      }
    }
    "2D Picture" <- w399
    "2D Picture 2" <- w399
    n228 = case shown="True" "OH BABY A TRIPLE" {
      tunnel: w397 -> [_ w410]
      frame False {
      }
      frame True {
        n229 = call <vilib>:"Application Directory.vi"() -> ("Application Directory"=w408:path)
        n230 = Build Path(base path=w408, name or relative path=w410) -> (appended path=w409:path)
        n231 = call "playsound.vi"("Sound File Path"=w409) -> ()  [unwired: 11 in]
      }
    }
    n232 = Wait (ms)(milliseconds to wait=u32 100) -> ()  [unwired: 1 out]
  }
  n233 = local write "Load"(TRUE ("Load")) -> ()
  n234 = call <vilib>:"Read PNG File.vi"("path to PNG file"=path "tote_stack_pics/bin.png" ("path to JPEG file")) -> ("image data"=w20:T66)  [unwired: 8 in, 2 out]
  n235 = while {
    tunnel: w22 -> [_]
    tunnel: w20 -> [_]
    stop <- FALSE stop-if-true
    n236 = case shown="True" "Useless Button" {
      tunnel: [60.0 w452] -> w436
      frame False {
      }
      frame True {
        n237 = Tick Count (ms)() -> (millisecond timer value=w457:u32)
        n238 = Quotient & Remainder(x=w457, y=u32 1000 ("milliseconds to wait")) -> (x-y*floor(x/y)=w461:u32)  [unwired: 1 out]
        n239 = Divide(x=w461, y=u32 1000 ("milliseconds to wait")) -> (x/y=w458:dbl)
        n240 = Multiply(x=6.283185307179586, y=w458) -> (x*y=w462:dbl)
        n241 = Sine(x=w462) -> (sin(x)=w456:dbl)
        n242 = Multiply(x=20.0, y=w456) -> (x*y=w454:dbl)
        n243 = Add(x=w454, y=40.0) -> (x+y=w452:dbl)
      }
    }
    n244 = local read "Robot Mode"() -> (w440:T4)
    n245 = local read "IMU Data"() -> (w448:T35)
    n246 = Unbundle By Name(w448) -> ("Data Valid?"=w444:bool)
    n247 = Equal?(x=w440, y=T4."Disconnected") -> (x = y?=w437:bool)
    n248 = Equal?(x=w440, y=T4."No Code") -> (x = y?=w438:bool)
    n249 = Or(x=w437, y=w438) -> (x .or. y?=w439:bool)
    n250 = Wait (ms)(milliseconds to wait=u32 50) -> ()  [unwired: 1 out]
    n251 = Or(x=w444, y=w439) -> (x .or. y?=w443:bool)
    n252 = control-ref of="Finger"() -> (w435:refnum<vi>)
    n253 = case shown="False" w443 {
      tunnel: [w464 u32 2829099 ("Base Color")] -> w445
      frame False {
        n254 = Tick Count (ms)() -> (millisecond timer value=w465:u32)
        n255 = Quotient & Remainder(x=w465, y=u32 1000 ("milliseconds to wait")) -> (x-y*floor(x/y)=w472:u32)  [unwired: 1 out]
        n256 = Divide(x=w472, y=u32 1000 ("milliseconds to wait")) -> (x/y=w469:dbl)
        n257 = Multiply(x=6.283185307179586, y=w469) -> (x*y=w474:dbl)
        n258 = Sine(x=w474) -> (sin(x)=w473:dbl)
        n259 = Absolute Value(x=w473) -> (abs(x)=w468:dbl)
        n260 = call "Interpolate RGB Color.vi"("Proportion"=w468, "Target Color"=u32 16711680, "Base Color"=u32 2829099) -> ("Result Color"=w464:u32)  [unwired: 8 in]
      }
      frame True {
      }
    }
    n261 = property on="Property Node" class="Bool (strict)"(reference=w435, "BoolText.FontSize"=w436) -> ()  [unwired: 1 in, 2 out]
    n262 = property on="Gyro" class="Knob (strict)"("BGColor"=w445) -> ("DigDisps[]"=w447:refnum<vi>[])  [unwired: 2 in, 2 out]
    n263 = Index Array(array=w447) -> (element=w446:refnum<vi>)  [unwired: 1 in]
    n264 = property class="DigNum"(reference=w446, "NumText.TextColor"=w445) -> ()  [unwired: 1 in, 2 out]
  }
